vi "Configure Experiment.vi"(8 "Error In":errorcluster, 9 "KH":T4 {"KH #" items=["A 1", "A 2", "A 3", "A 4", "A 5", "A 6", "A 7", "A 8"]}, 10 "Lockin":T6 {"Label" items=["", "I+", "I-", "V1+", "V1-", "V2+", "V2-", "V3+", "V3-", "V4+", "V4-", "dV1", "dV2", "dV3", "Vsg", "Vbg", "Vtg"]}) -> (0 "Error Out":errorcluster)   [LabVIEW 2019, in "Control Experiment.lvclass"]
doc: "Use this VI to help configure your experiment.\n1. Configure the Electrode control to show which electrode is connected to which lockin channel;\n2. Choose a Label for each electrode to configure Krohn Hite amplifier automatically\n3. Easily set all Krohn Hite channels to be \"all ground\" or \"all differential\" mode\n4. Fill out information about you and your device in the lower left corner\n5. When you are finished, or when you want to update the amplifiers, click the \"CREATE OUTPUT\" button located in upper right. Clicking this button will set the amplifiers, and write information to a functional global variable that you can easily read from elsewhere in your program"
uses:
  Control Experiment.lvclass
  Typedefs/KH Mode-enum.ctl
  <userlib>/LevyLab/Krohn Hite 7008/KH7008/typedefs/Input--Enum.ctl
  <userlib>/LevyLab/Krohn Hite 7008/KH7008/typedefs/gain--enum.ctl
  <userlib>/LevyLab/Krohn Hite 7008/KH7008/typedefs/shunt--enum.ctl
  <userlib>/LevyLab/Krohn Hite 7008/KH7008/typedefs/allChannelProperties--Array.ctl
  <userlib>/LevyLab/Krohn Hite 7008/KH7008/typedefs/channelProperties--Cluster.ctl
  <userlib>/LevyLab/Krohn Hite 7008/KH7008/typedefs/channel--numeric.ctl
  <userlib>/LevyLab/Krohn Hite 7008/KH7008/typedefs/couple--Enum.ctl
  <userlib>/LevyLab/Krohn Hite 7008/KH7008/typedefs/Filter--Enum.ctl
  <userlib>/LevyLab/Configuration/Configuration.lvclass
  Typedefs/UI Controls --cluster.ctl
  Typedefs/Instruments--cluster.ctl
  Typedefs/Instrument Types--enum.ctl
  Transport Server/Inst.Transport/Inst.Transport.lvclass
  C:/Program Files/National Instruments/LabVIEW 2019/vi.lib/JKI/JKI SMO/SMO/SMO.lvclass
  C:/Program Files/National Instruments/LabVIEW 2019/user.lib/LevyLab/Instrument Framework/Instrument/Instrument.lvclass
  Transport/Transport.lvclass
  Control Experiment.lvclass/Control Experiment.ctl
  <vilib>/JKI/JKI SMO/SMO/SMO.lvclass/SMO.ctl
  Transport Server/Inst.Transport/Inst.Transport.lvclass/Inst.Transport.ctl
  Typedefs/Instrument Classes--cluster.ctl
  <userlib>/LevyLab/Instrument Framework/Instrument Types/Lockin/Instrument.LockinAPI.lvclass
  <userlib>/LevyLab/Instrument Framework/Instrument Types/Amplifier/Instrument.Amplifier.lvclass
  <userlib>/LevyLab/Instrument Framework/Instrument Types/Cryostat/Instrument.Cryostat.lvclass
  <userlib>/LevyLab/Instrument Framework/Instrument Types/CBridge/Instrument.CBridge.lvclass
  <userlib>/LevyLab/Instrument Framework/Instrument Types/Delay Line/Instrument.DelayLine.lvclass
  <userlib>/LevyLab/Instrument Framework/Instrument Types/Strain/Instrument.Strain.lvclass
  <userlib>/LevyLab/Instrument Framework/Instrument Types/VNA/Instrument.VNA.lvclass
  <userlib>/LevyLab/Instrument Framework/Instrument Types/VSource/Instrument.VSource.lvclass
  <userlib>/LevyLab/Krohn Hite 7008/Inst.Krohn-Hite-7008/Inst.Krohn-Hite-7008.lvclass
  C:/Program Files/National Instruments/LabVIEW 2019/user.lib/LevyLab/Instrument Framework/Instrument Types/Amplifier/Instrument.Amplifier.lvclass
  Typedefs/Control Experiment JSON--cluster.ctl
  b06a41f5-2f73-4e7a-a8dc-a6b31f20112d.vi
  <vilib>/JKI/JKI SMO/SMO/Private/ReftoDVR--SMO.vi
  <vilib>/JDP Science/JSONtext/Variant to JSON Text.vi
  <vilib>/JDP Science/JSONtext/LVClass Serializer/JSONtext LVClass Serializer.lvclass
  <vilib>/ErrorRing/Error Ring.xnode
  <userlib>/LevyLab/Krohn Hite 7008/KH7008/KH7008.lvlib
  <vilib>/JKI/JKI SMO/SMO/SMO.lvclass
  <userlib>/LevyLab/Instrument Framework/Instrument/Instrument.lvclass
  <vilib>/JKI/JKI SMO/URI Parsing/URI.lvlib
panel:
  in  "I'm Finished Taking Data!":bool
  out "State":string
  in  "Create Output":bool
  in  "String":string
  out "Values have changed":bool=TRUE
  in  "OK":bool
  out "Control Experiment":refnum<class "Control Experiment.lvclass">
  in  "C.E.":refnum<class "Control Experiment.lvclass">
  in  "Tab Control":enum32{"Input", "Output", "Configuration"}(tab)
  out "KH S/N":string
  out "MCL S/N":string
  in  "Transport Server":bool
  in  "Open KH7008":bool
  in  "Open Lockin":bool
  out "Lockin?":bool
  out "KH?":bool
  out "Transport?":bool
  in  "KH Chassis":i32 caption="AI Channels"
  in  "Type":u16(ring) items=["AFM", "EBL", "Cryo"]
  in  "Instrument Configuration":bool
  out "Configured Instruments":string
  in  "DC Coupled":bool=TRUE
  in  "BW Filter":bool=TRUE
  in  "AO Channels":u32=8
  in  "Gain":dbl[](array[numeric])=[1.0, 1.0, 1.0, 1.0, 1.0, 1.0, 1.0, 1.0, 1.0, 1.0, 1.0, 1.0, 1.0, 1.0, 1.0, 1.0]
  in  "AI Channels":u32=8
  in  "KH Configuration":T7(radio)
  in  "Default Resistor":T3=enum."5k"
  in  "Description":string
  in  "Sample (SAXXXX)":string
  in  "Device":string
  in  "Station":u16(ring) items=["CF900", "MNK", "PPMS (sim)", "Montana", "PPMS1", "PPMS2", "PPMS3", "OptiCool", "PPMS-W-1"]
  in  "User":u16(ring) items=["Jeremy", "Patrick", "Guanglei", "Juliana", "Ranjani", "Ahmed", "Yuhao", "Pubudu", "Sayanwita", "Aswini", "Aria", "Miles", "Bohao", "Sakshi"]
  in  "non KH":T8 {"Labels 2" items=["", "I+", "I-", "V1+", "V1-", "V2+", "V2-", "V3+", "V3-", "V4+", "V4-", "dV1", "dV2", "dV3", "Vsg", "Vbg", "Vtg"]}
  out "Device Folder":path=path "D:/Data/MNK/SA40178.20210125" caption="(\\base path\\project\\device\\ )"
  in  "Path":path=path "C:/temp" caption="Path (Typ. C:\\Users\\voodoo\\Nextcloud2\\Shared\\Instrument\\)"
  out "Comments":string
  out "JSON String":string
  in  "Label Strings":string
  # "Lockin"
  # "Krohn-Hite"
  # "Other"
  # "Channel and Chassis Configuration"
  # "Device and Project Description"
  # "Instrument Configuration"
  # "Apps"
  # "Path Configuration"
  # "Instructions: This application is used to configure your experiment\n\n1. Configure the Electrode control to show which electrode is connected to which lockin\n2. Choose a Label* for each electrode to configure Krohn Hite amplifier automatically\n3. Easily set all Krohn Hite channels to be \"all ground\" or \"all differential\" mode\n4. Fill out information about you and your device in the lower left corner\n5. When you are finished, or when you want to update the amplifiers, click the \"CONFIRM\" button located in upper right. Clicking this button will set the amplifiers and write information to a file that you can easily read from elsewhere in your program\n\n*If you want to have new labels for the \"Labels\" field you can type them below. Acceptable keywords are I, Vsg, Vbg, Vtg, dV, V, along with numeric indicies and +/-. Examples: V1+, V1-, dV1"
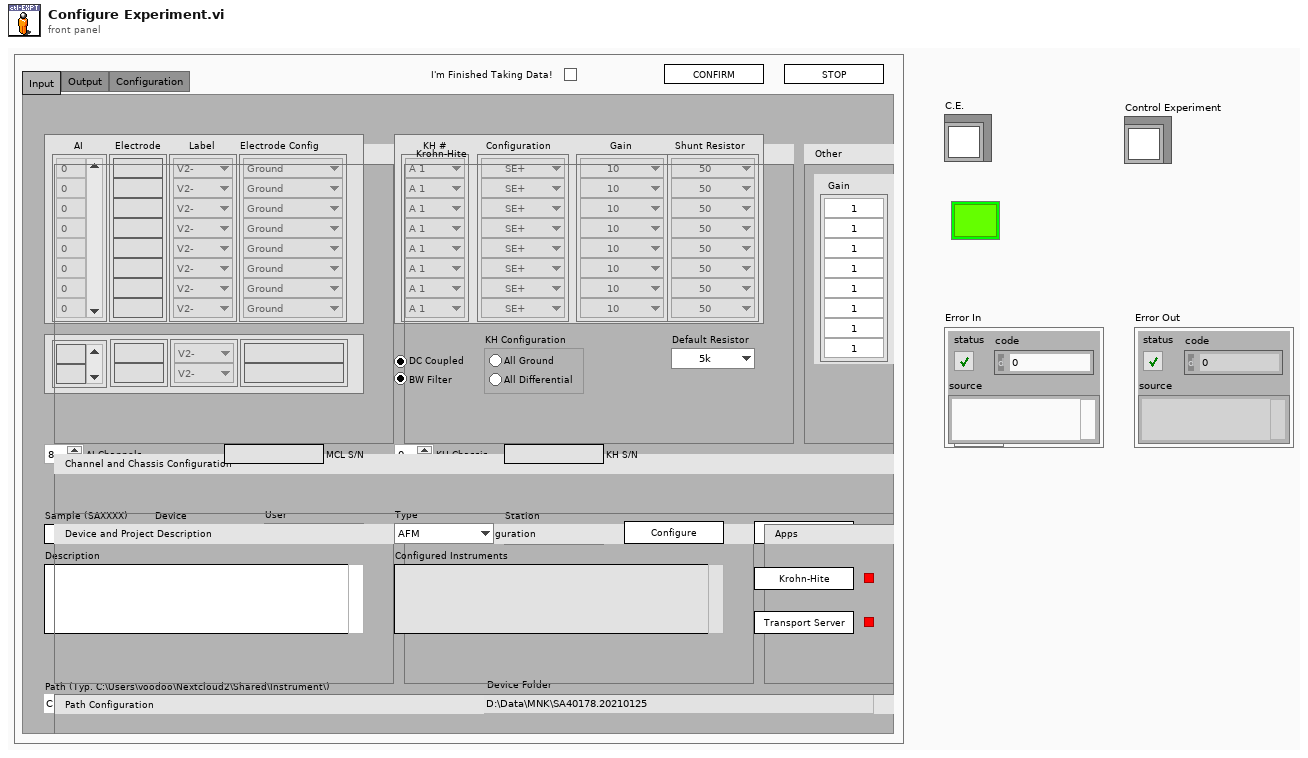
[diagram p1: front panel]
types:
  T1 = typedef "KH7008.lvlib/Input--Enum.ctl" = enum16{"OFF", "SE+", "SE-", "DIFF"}
  T2 = typedef "KH7008.lvlib/gain--enum.ctl" = enum16{"1", "10", "100", "1000"}
  T3 = typedef "KH7008.lvlib/shunt--enum.ctl" = enum16{"Open", "50", "500", "5k", "50k", "10M"}
  T4 = cluster{"KH #":u16[], "KH Configuration":T1[], "KH Gain":T2[], "KH Shunt Resistor":T3[]}
  T5 = typedef "Control Experiment.lvclass/KH Mode-enum.ctl" = enum16{"Ground", "Current", "Voltage (SE)", "Voltage (Diff)", "Gate"}
  T6 = cluster{"AI":u32[], "Electrode":string[], "Label":u16[], "Electrode Config":T5[]}
  T7 = enum32{"No Selection", "All Ground", "All Differential"}
  T8 = cluster{"Scroll Bar":string[], "Electrodes 2":string[], "Labels 2":u16[], "unused":string[]}
  T9 = enum32{"invalid app kind", "Development System", "Run Time System", "Student Edition", "Embedded LabVIEW", "Evaluation", "Custom"}
  T10 = enum32{"Bad", "Idle", "Run top level", "Running"}
  T11 = typedef "Control Experiment.lvclass/Instrument Classes--cluster.ctl" = cluster{"DAQ":refnum<class "Instrument.LockinAPI.lvclass">, "Amplifier":refnum<class "Instrument.Amplifier.lvclass">, "Temperature":refnum<class "Instrument.Cryostat.lvclass">, "Magnet":refnum<class "Instrument.Cryostat.lvclass">, "Rotator":refnum<class "Instrument.Cryostat.lvclass">, "Level":refnum<class "Instrument.Cryostat.lvclass">, "Capacitance":refnum<class "Instrument.CBridge.lvclass">, "Delay Line":refnum<class "Instrument.DelayLine.lvclass">, "Strain Cell":refnum<class "Instrument.Strain.lvclass">, "VNA":refnum<class "Instrument.VNA.lvclass">, "Source":refnum<class "Instrument.VSource.lvclass">}
  T12 = enum32{"Invalid", "Standard", "Closed", "Hidden", "Minimized", "Maximized"}
  T13 = typedef "KH7008.lvlib/channelProperties--Cluster.ctl" = cluster{"channel":T14, "gain":T2, "input":T1, "shunt":T3, "couple":T15, "filter":T16}
  T14 = typedef "KH7008.lvlib/channel--numeric.ctl" = u16
  T15 = typedef "KH7008.lvlib/couple--Enum.ctl" = enum16{"AC", "DC"}
  T16 = typedef "KH7008.lvlib/Filter--Enum.ctl" = enum16{"OFF", "ON"}
  T17 = typedef "Control Experiment.lvclass/Experiment Description--cluster.ctl" = cluster{"User":string, "Device":string, "Device Path":path, "Device Description":string, "Experiment Path":path, "Experiment Description":string, "Instrument":string, "Instruments":T18[], "Sweep":cluster{"key":string, "value":variant}[]}
  T18 = typedef "Control Experiment.lvclass/Instruments--cluster.ctl" = cluster{"class path":path, "Address":string, "Type":T19}
  T19 = typedef "Control Experiment.lvclass/Instrument Types--enum.ctl" = enum16{"DAQ", "Amplifier", "Temperature", "Magnet", "Rotator", "Level", "Capacitance", "Delay Line", "Strain Cell", "VNA", "Source"}
  T20 = typedef "Control Experiment.lvclass/Wiring Description--cluster.ctl" = cluster{"Lockin Ch":i32[], "KH":cluster{"Electrodes":string[], "Labels":string[]}, "not KH":cluster{"Electrodes":string[], "Labels":string[]}}
  T21 = typedef "KH7008.lvlib/allChannelProperties--Array.ctl" = T13[]
  T22 = typedef "Control Experiment.lvclass/UI Controls --cluster.ctl" = cluster{"Sample":string, "Device":string, "Username":string, "Description":string, "Default Path":path, "Instrument":string, "Station Type":string, "KH All Buttons":enum32{"No Selection", "All Ground", "All Differential"}, "Lockin":cluster{"AI":u32[], "Electrode":string[], "Label":u16[], "Electrode Config":T5[], "AI Channels":u32}, "KH":cluster{"KH #":enum16{"A 1", "A 2", "A 3", "A 4", "A 5", "A 6", "A 7", "A 8", "B 1", "B 2", "B 3", "B 4", "B 5", "B 6", "B 7", "B 8", "none"}[], "KH Configuration":T1[], "KH Gain":T2[], "KH Shunt Resistor":T3[], "Filter":bool, "DC Coupled":bool, "KH Chassis":i32}, "non KH":cluster{"Scroll Bar":string[], "Electrodes 2":string[], "Labels 2":u16[], "unused":string[]}, "Instrument Types":T18[]}
  T23 = cluster{"Core":cluster{"Current VI Reference":refnum<vi>, "Close Panel on Exit?":bool}, "C.E.":refnum<class "Control Experiment.lvclass">, "Experiment":T17, "Wiring Configuration":T20, "Channel Settings":cluster{"Channel Setting":T21}[], "KH Configuration":enum32{"No Selection", "All Ground", "All Differential"}, "Lockin":cluster{"AI":u32[], "Electrode":string[], "Label":u16[], "Electrode Config":T5[]}, "KH":cluster{"KH #":u16[], "KH Configuration":T1[], "KH Gain":T2[], "KH Shunt Resistor":T3[]}, "non KH":cluster{"Scroll Bar":string[], "Electrodes 2":string[], "Labels 2":u16[], "unused":string[]}, "UI":T22, "Config":refnum<class "Configuration.lvclass">, "Transport":refnum<class "Transport.lvclass">, "Transport-Server":refnum<class "Inst.Transport.lvclass">, "top level?":bool, "Instruments OK?":bool}
  T24 = typedef "SMO.lvclass/SMOState --Enum.ctl" = enum16{"unknown", "Created", "Started", "Stopped"}
  T25 = typedef "Inst.Transport.lvclass/UI State--enum.ctl" = enum16{"unknown", "Opened", "Closed"}
  T26 = cluster{"Current VI Reference":refnum<vi>, "Close Panel on Exit?":bool}
  T27 = typedef "SMO.lvclass/Public Events.ctl" = cluster{"Error":refnum<user-event>, "State":refnum<user-event>, "Reserve State":refnum<user-event>}
  T28 = typedef "Inst.Transport.lvclass/PublicEvents--Cluster.ctl" = cluster{"UI State":refnum<user-event>}
  T29 = cluster{"AI":u32[], "Electrode":string[], "Label":u16[], "Electrode Config":T5[], "AI Channels":u32}
  T30 = cluster{"KH #":enum16{"A 1", "A 2", "A 3", "A 4", "A 5", "A 6", "A 7", "A 8", "B 1", "B 2", "B 3", "B 4", "B 5", "B 6", "B 7", "B 8", "none"}[], "KH Configuration":T1[], "KH Gain":T2[], "KH Shunt Resistor":T3[], "Filter":bool, "DC Coupled":bool, "KH Chassis":i32}
  T31 = enum16{"A 1", "A 2", "A 3", "A 4", "A 5", "A 6", "A 7", "A 8", "B 1", "B 2", "B 3", "B 4", "B 5", "B 6", "B 7", "B 8", "none"}[]
  T32 = typedef "Control Experiment.lvclass/Control Experiment JSON--cluster.ctl" = cluster{"Device":cluster{"Device":string, "User":string, "Time":string, "Computer Name":string}, "Wiring":cluster{"Lockin Ch":u32[], "KH Electrodes":string[], "KH Labels":string[], "Other Electrodes":string[], "Other Labels":string[]}}
  T33 = typedef "Instrument.lvlib/Instrument.lvclass/Instrument.IDN--cluster.ctl" = cluster{"vendor":string, "model":string, "serial":string, "firmware":string}
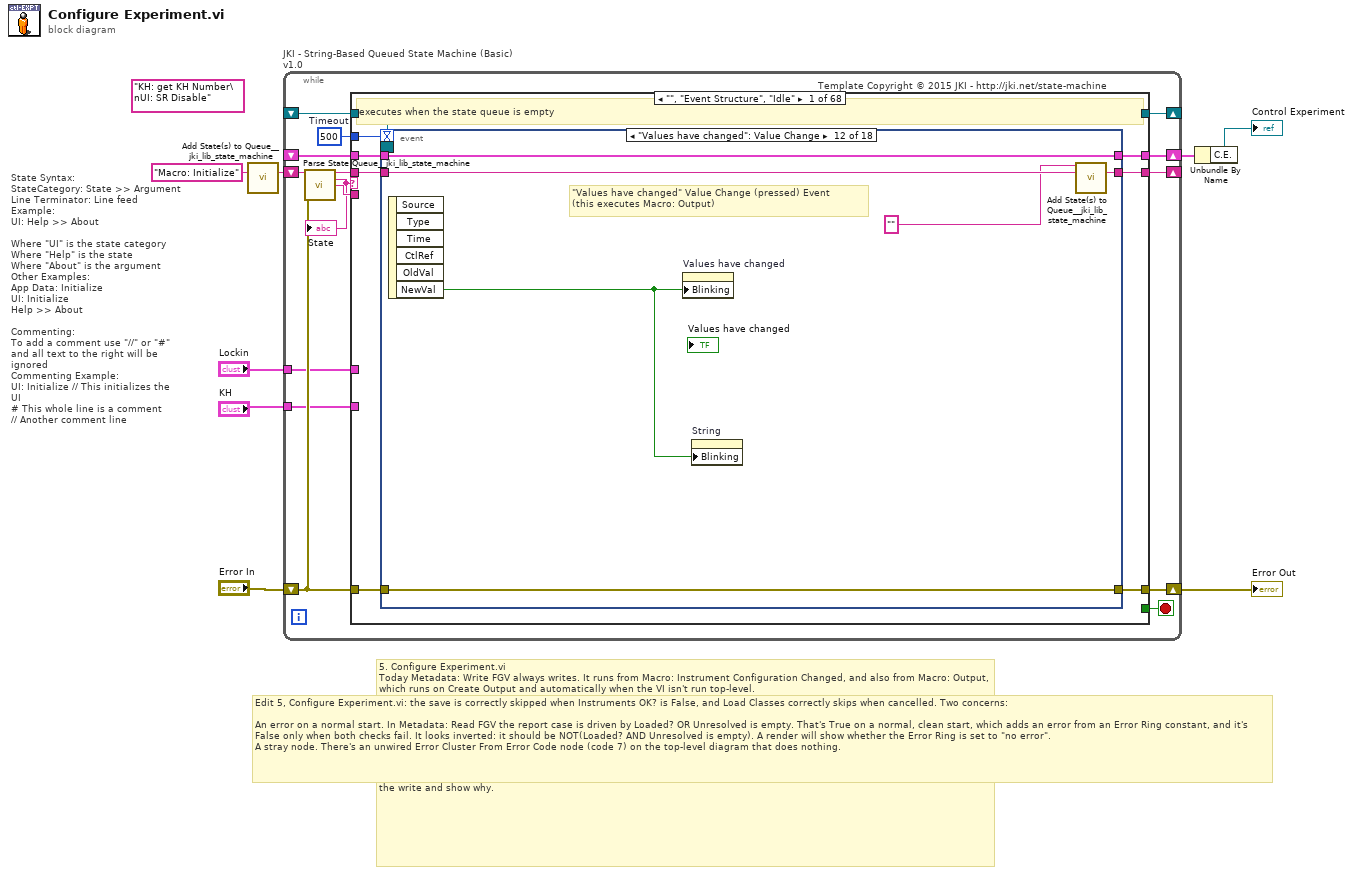
[diagram p0: block diagram]
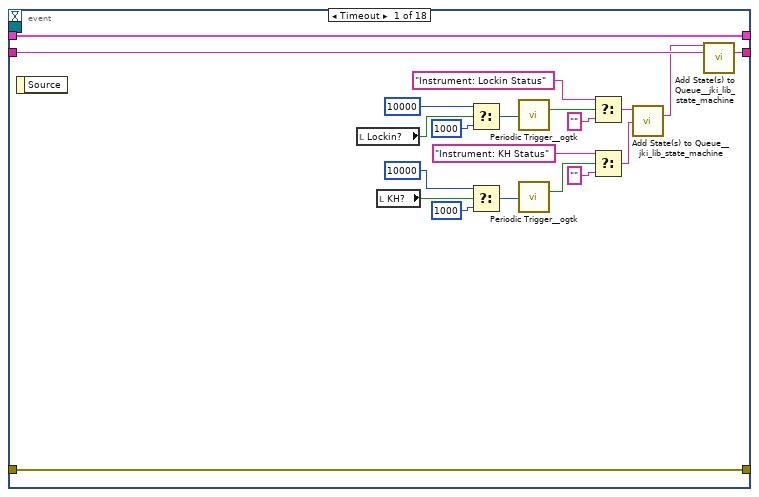
[diagram p2: hidden frame]
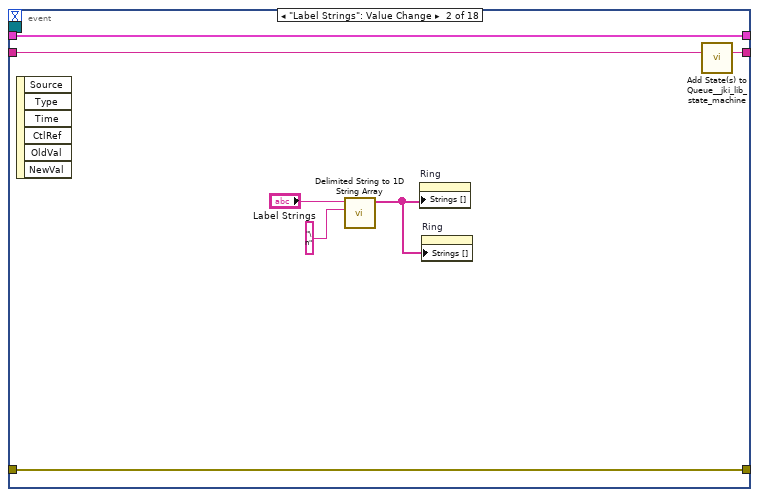
[diagram p3: hidden frame]
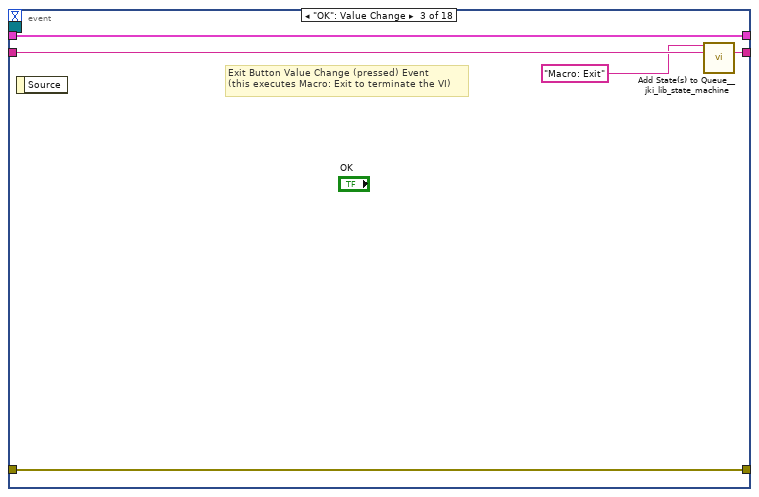
[diagram p4: hidden frame]
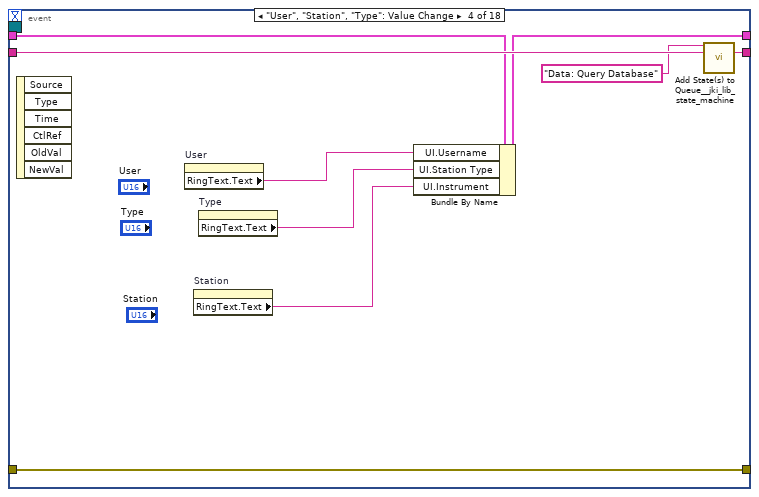
[diagram p5: hidden frame]
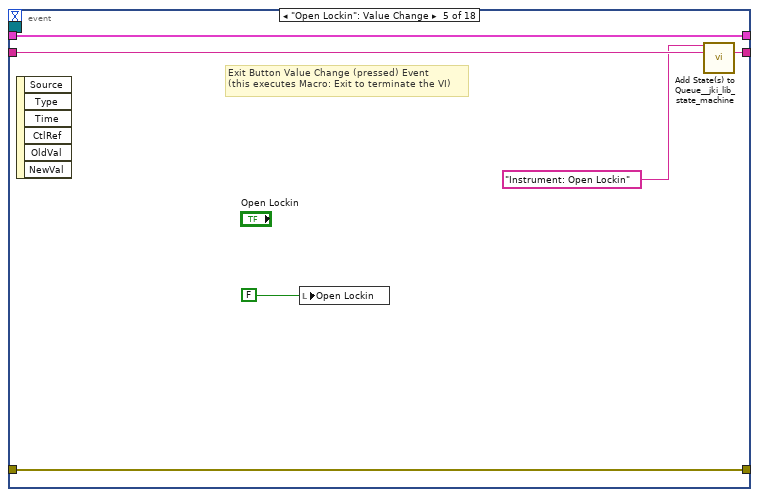
[diagram p6: hidden frame]
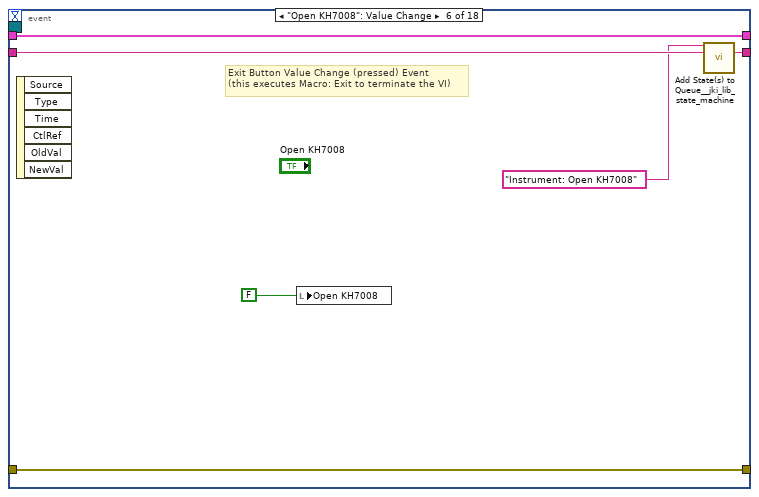
[diagram p7: hidden frame]
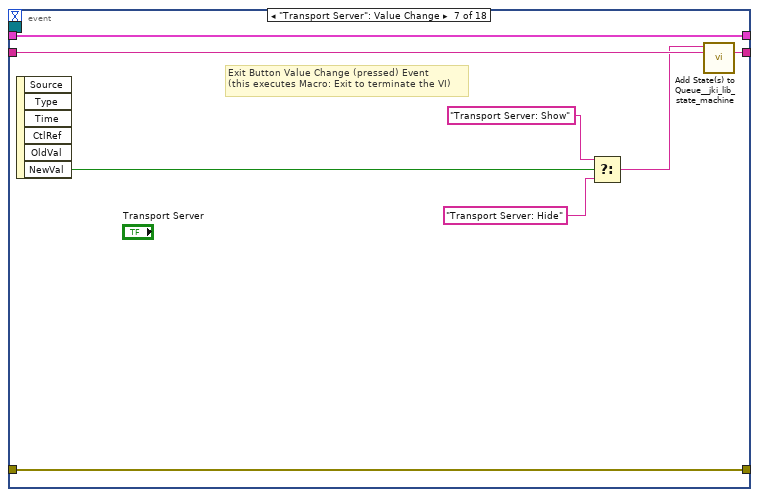
[diagram p8: hidden frame]
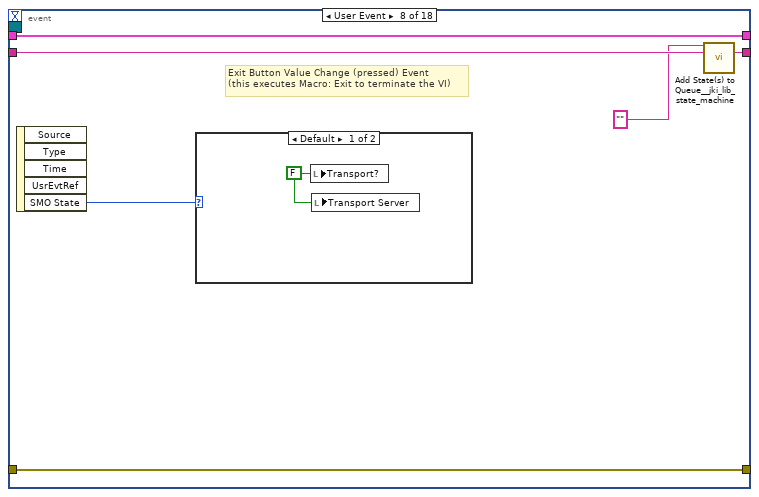
[diagram p9: hidden frame]
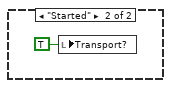
[diagram p10: hidden frame]
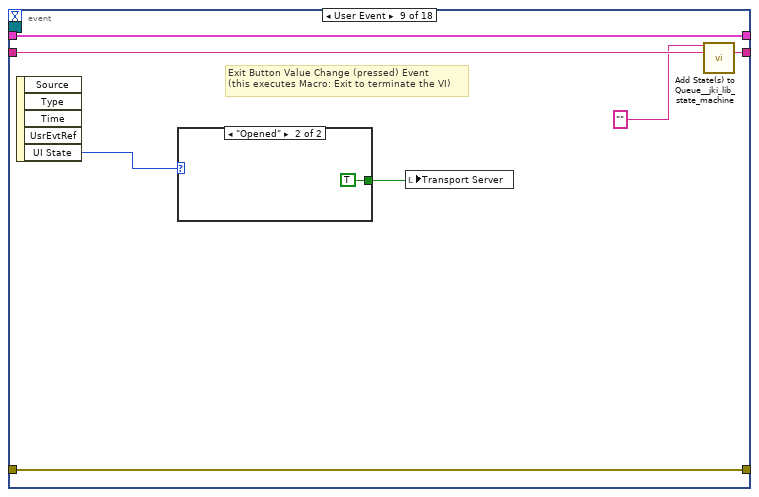
[diagram p11: hidden frame]
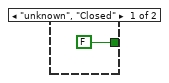
[diagram p12: hidden frame]
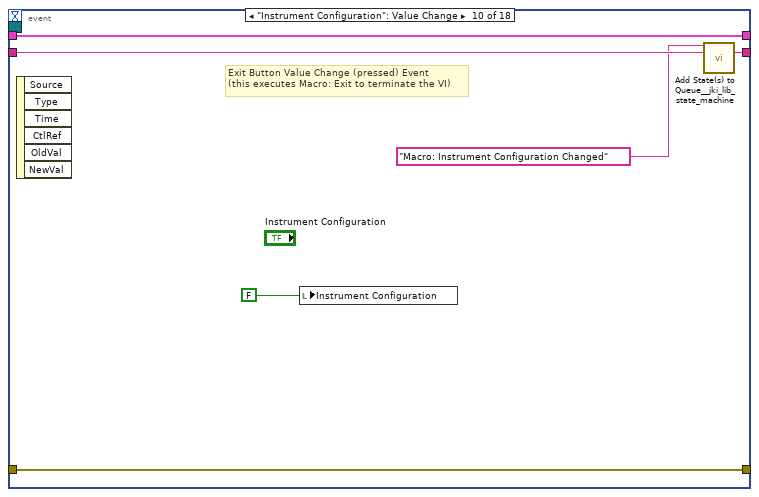
[diagram p13: hidden frame]
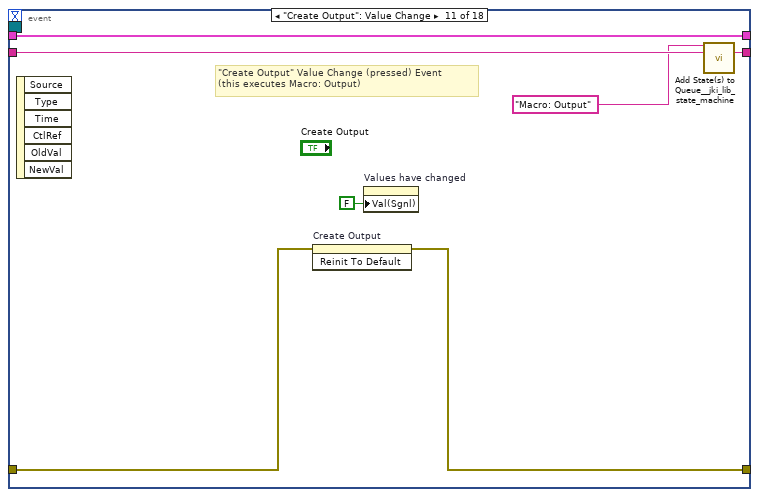
[diagram p14: hidden frame]
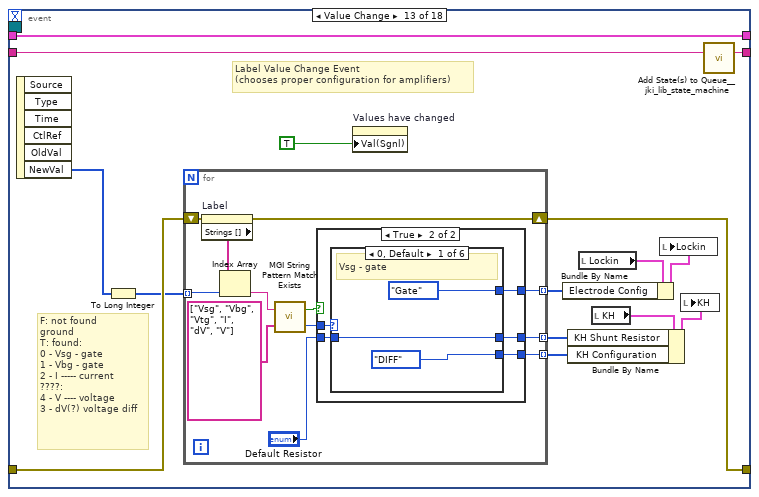
[diagram p15: hidden frame]
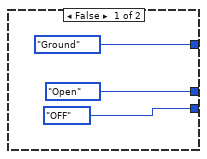
[diagram p16: hidden frame]
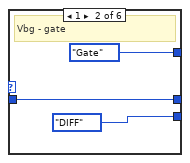
[diagram p17: hidden frame]
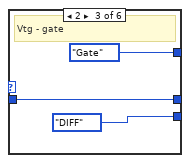
[diagram p18: hidden frame]
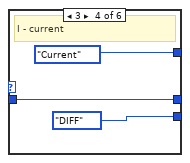
[diagram p19: hidden frame]
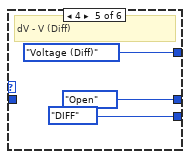
[diagram p20: hidden frame]
diagram:
  (unwired) "KH: get KH Number\nUI: SR Disable" ("State(s) in Front (\"\")")
  # "Edit 5, Configure Experiment.vi: the save is correctly skipped when Instruments OK? is False, and Load Classes correctly skips when cancelled. Two concerns:\n\nAn error on a normal start. In Metadata: Read FGV the report case is driven by Loaded? OR Unresolved is empty. That's True on a normal, clean start, which adds an error from an Error Ring constant, and it's False only when both checks fail. It looks inverted: it should be NOT(Loaded? AND Unresolved is empty). A render will show whether the Error Ring is set to \"no error\".\nA stray node. There's an unwired Error Cluster From Error Code node (code 7) on the top-level diagram that does nothing."
  # "5. Configure Experiment.vi\nToday Metadata: Write FGV always writes. It runs from Macro: Instrument Configuration Changed, and also from Macro: Output, which runs on Create Output and automatically when the VI isn't run top-level.\n\n1. Add a boolean Instruments OK? to the data cluster.\n2. Metadata: Read FGV: set Instruments OK? = Loaded? AND Unresolved on load is empty. If there's no saved configuration or entries are unresolved, tell the user: error 7 means \"no saved configuration\"; show other errors as they are.\n3. Instruments: Load Classes:\na. If Cancelled? is True, leave C.E. and Instruments OK? unchanged.\nb. Otherwise set Instruments OK? = Unresolved is empty.\n4. Metadata: Write FGV: put the Control Experiment FGV.vi (write) call inside a Case on Instruments OK?. When it is False, skip the write and show why."
  # "State Syntax:\nStateCategory: State >> Argument\nLine Terminator: Line feed\nExample:\nUI: Help >> About\n\nWhere \"UI\" is the state category\nWhere \"Help\" is the state\nWhere \"About\" is the argument\nOther Examples:\nApp Data: Initialize\nUI: Initialize\nHelp >> About\n\nCommenting:\nTo add a comment use \"//\" or \"#\" and all text to the right will be ignored\nCommenting Example:\nUI: Initialize // This initializes the UI\n# This whole line is a comment\n// Another comment line"
  n1 = call <vilib>:"Add State(s) to Queue__jki_lib_state_machine.vi"("State(s) in (\"\")"="Macro: Initialize") -> ("States Out"=w8:string)  [unwired: 14 in]
  n2 = while "JKI - String-Based Queued State Machine (Basic) v1.0" {
    shift-right: [w17] -> w6
    shift-left: _ -> [w16]
    shift-right: [w20] -> w2
    shift-left: "Error In" -> [w14]
    shift-right: [w19] -> _
    shift-left: w8 -> [w21]
    tunnel: "Lockin" -> [w13]
    tunnel: "KH" -> [w12]
    shift-right: [w10] -> _
    shift-left: _ -> [w9]
    stop <- w18 stop-if-true
    w15 = 500  # Timeout
    # "Template Copyright © 2015 JKI - http://jki.net/state-machine"
    n3 = call <vilib>:"Parse State Queue__jki_lib_state_machine.vi"("State Queue"=w21, "Error In (no error)"=w14) -> ("Remaining States"=w23:string, "Current State"=w11:string, "Arguments"=w22:string)  [unwired: 11 in]
    "State" <- w11
    n4 = case shown="\"\", \"Event Structure\", \"Idle\"" w11 {
      selector: w11 -> [_ _ w234 _ _ _ _ _ _ _ _ _ _ _ _ _ _ _ _ _ _ _ _ _ _ _ _ _ _ _ _ _ _ _ _ _ _ _ _ _ _ _ _ _ _ _ _ _ _ _ _ _ _ _ _ _ _ _ _ _ _ _ _ _ _ _ _ _]
      tunnel: w23 -> [w31 w232 w238 w257 w264 w270 w275 w295 w307 w323 w355 w362 w392 w397 w410 w416 w421 w443 w474 w494 w530 w542 w569 w585 w600 w621 w627 w639 w647 w654 w660 w666 w671 w684 w703 w728 w788 w841 w851 w863 w885 w893 w914 w927 w942 w976 w1068 w1113 w1134 w1150 w1161 w1172 w1191 w1227 w1255 w1287 w1293 w1298 w1309 w1318 w1327 w1336 w1344 w1352 w1357 w1373 w1378 w1386]
      tunnel: w22 -> [_ _ _ _ _ _ _ _ _ _ _ _ _ _ _ _ _ _ _ _ w525 w536 _ _ _ _ _ _ _ _ _ _ _ _ _ _ _ _ _ _ _ _ _ _ _ _ _ _ _ _ _ _ _ _ _ _ _ _ _ _ _ _ _ _ _ _ _ w1381]
      tunnel: w16 -> [w29 w229 w236 w248 w261 w268 w272 _ w302 w309 w335 w359 w384 w394 w408 w414 w418 w436 w463 w492 w528 w538 w566 w582 w598 w618 w624 w636 w645 w651 w657 w663 w668 w680 w699 w726 w786 w839 w847 w861 w871 w891 w908 w924 w940 w968 w1063 w1108 w1130 w1147 w1159 w1169 w1182 w1222 w1250 w1285 w1291 w1295 w1306 w1311 w1323 w1330 w1341 w1349 w1354 w1371 w1375 w1383]
      tunnel: [w28 w230 w240 w254 errorcluster {"status"=FALSE, "code"=0, "source"=""} ("error out") w267 w273 w292 w305 w320 w345 w360 w390 w395 w404 w411 w419 w424 w472 w487 w526 w539 w567 w583 w590 w619 w625 w637 w643 w652 w658 w664 w669 w682 w701 w719 w781 w834 w844 w854 w867 w889 w902 w925 w932 w967 w1065 w1106 w1131 w1148 w1154 w1170 w1189 w1225 w1253 w1283 w1289 w1296 w1300 w1314 w1319 w1333 w1340 w1348 w1355 w1363 w1376 w1384] -> w20
      tunnel: w14 -> [w27 w230 w239 w254 w260 w267 w273 w292 w305 w321 w346 w357 w390 w395 w403 w412 w419 w441 w472 w487 w527 w540 w567 w583 w591 w619 w625 w637 w643 w652 w658 w664 w669 w682 w701 w716 w778 w835 w844 w855 w873 w888 w911 w925 w930 w967 w1058 w1105 w1127 w1148 w1156 w1170 w1189 w1225 w1253 w1284 w1290 w1296 w1302 w1313 w1320 w1332 w1339 w1347 w1355 w1364 w1376 w1384]
      tunnel: [w30 w231 w237 w256 w263 w269 w274 w294 w306 w322 w354 w361 w391 w396 w409 w415 w420 w442 w473 w493 w529 w541 w568 w584 w599 w620 w626 w638 w646 w653 w659 w665 w670 w683 w702 w727 w787 w840 w850 w862 w884 w892 w913 w926 w941 w975 w1067 w1112 w1133 w1149 w1160 w1171 w1190 w1226 w1254 w1286 w1292 w1297 w1308 w1317 w1326 w1335 w1343 w1351 w1356 w1372 w1377 w1385] -> w19
      tunnel: [_ _ _ _ _ TRUE _ _ _ _ _ _ _ _ _ _ _ _ _ _ _ _ _ _ _ _ _ _ _ _ _ _ _ _ _ _ _ _ _ _ _ _ _ _ _ _ _ _ _ _ _ _ _ _ _ _ _ _ _ _ _ _ _ _ _ _ _ _] -> w18
      tunnel: [w26 w229 w236 w255 w261 w268 w272 w293 w301 w308 w336 w359 w385 w394 w408 w414 w418 w436 w463 w492 w528 w538 w566 w582 w598 w618 w624 w636 w645 w651 w657 w663 w668 w681 w700 w712 w772 w838 w846 w860 w872 w891 w909 w924 w939 w974 w1066 w1108 w1132 w1147 w1158 w1169 w1183 w1223 w1251 w1285 w1291 w1295 w1307 w1312 w1324 w1331 w1342 w1350 w1354 w1371 w1375 w1383] -> w17
      tunnel: w15 -> [w25 _ _ _ _ _ _ _ _ _ _ _ _ _ _ _ _ _ _ _ _ _ _ _ _ _ _ _ _ _ _ _ _ _ _ _ _ _ _ _ _ _ _ _ _ _ _ _ _ _ _ _ _ _ _ _ _ _ _ _ _ _ _ _ _ _ _ _]
      tunnel: w13 -> [_ _ _ _ _ _ _ w281 _ _ _ _ _ _ _ _ _ _ _ _ _ _ _ _ _ _ _ _ _ _ _ _ _ _ _ _ _ _ _ _ _ _ _ _ _ _ _ _ _ _ _ _ _ _ _ _ _ _ _ _ _ _ _ _ _ _ _ _]
      tunnel: w12 -> [_ _ _ _ _ _ _ w280 _ _ _ _ _ _ _ _ _ _ _ _ _ _ _ _ _ _ _ _ _ _ _ _ _ _ _ _ _ _ _ _ _ _ _ _ _ _ _ _ _ _ _ _ _ _ _ _ _ _ _ _ _ _ _ _ _ _ _ _]
      tunnel: [w24 w228 w233 w245 w258 w265 w271 w277 w296 w319 w324 w356 w363 w393 w402 w413 w417 w433 w445 w486 w524 w535 w565 w570 w597 w617 w622 w628 w640 w649 w655 w661 w667 w672 w687 w710 w771 w831 w842 w852 w864 w887 w907 w923 w928 w956 w1047 w1098 w1121 w1146 w1153 w1168 w1188 w1224 w1252 w1282 w1288 w1294 w1305 w1310 w1322 w1328 w1338 w1346 w1353 w1362 w1374 w1382] -> w10
      tunnel: w9 -> [w24 w228 w233 w245 w258 w265 w271 w277 w296 w319 w324 w356 w363 w393 _ w413 w417 w433 w445 w486 w524 w535 w565 w570 w597 w617 w622 w628 w640 w649 w655 w661 w667 w672 w687 w710 w771 w831 w842 w852 w864 w887 w907 w923 w928 w956 w1047 w1098 w1121 w1146 w1153 w1168 w1188 w1224 w1252 w1282 w1288 w1294 w1305 w1310 w1322 w1328 w1338 w1346 w1353 w1362 w1374 w1382]
      frame "", "Event Structure", "Idle" {
        # "executes when the state queue is empty"
        n5 = event shown="[11] \"Values have changed\": Value Change" {
          selector: w24 -> [_ _ _ _ _ _ _ _ _ _ _ _ _ _ _ _ _ _]
          dyn-events: _ -> [_ _ _ _ _ _ _ _ _ _ _ _ _ _ _ _ _ _]
          timeout: w25 -> [_ _ _ _ _ _ _ _ _ _ _ _ _ _ _ _ _ _]
          tunnel: w31 -> [w52 w57 w64 w73 w79 w85 w93 w99 w108 w116 w123 w129 w144 w184 w189 w207 w213 w227]
          tunnel: [w51 w59 w63 w72 w78 w84 w92 w98 w107 w115 w122 w128 w143 w184 w188 w206 w215 w226] -> w30
          tunnel: w29 -> [w49 w58 w61 w68 w76 w82 w90 w96 w105 w113 w121 w127 w142 w185 w190 w205 w216 w224]
          tunnel: [w50 w56 w62 w71 w77 w83 w91 w97 w106 w114 w118 w125 w133 w186 w191 w208 w212 w225] -> w28
          tunnel: w27 -> [w50 w56 w62 w71 w77 w83 w91 w97 w106 w114 w119 w125 w140 w186 w191 w208 w212 w225]
          tunnel: [w49 w58 w61 w69 w76 w82 w90 w96 w105 w113 w121 w127 w142 w185 w190 w205 w216 w224] -> w26
          event Timeout {
            n6 = event-data() -> ()  [unwired: 1 in, 1 out]
            n7 = local read "Lockin?"() -> (w36:bool)
            n8 = local read "KH?"() -> (w37:bool)
            n9 = Select(t=u32 10000 ("time (ms)"), s=w36, f=u32 1000) -> (s? t:f=w39:u32)
            n10 = Select(t=u32 10000 ("time (ms)"), s=w37, f=u32 1000) -> (s? t:f=w38:u32)
            n11 = call <userlib>:"Periodic Trigger__ogtk.vi"("time (ms)"=w39) -> ("Triggered"=w33:bool)  [unwired: 12 in, 2 out]
            n12 = call <userlib>:"Periodic Trigger__ogtk.vi"("time (ms)"=w38) -> ("Triggered"=w32:bool)  [unwired: 12 in, 2 out]
            n13 = Select(t="Instrument: Lockin Status", s=w33, f="") -> (s? t:f=w43:string)
            n14 = Select(t="Instrument: KH Status", s=w32, f="") -> (s? t:f=w46:string)
            n15 = call <vilib>:"Add State(s) to Queue__jki_lib_state_machine.vi"("State(s) in Front (\"\")"=w43, "State(s) at Back (\"\")"=w46) -> ("States Out"=w42:string)  [unwired: 13 in]
            n16 = call <vilib>:"Add State(s) to Queue__jki_lib_state_machine.vi"("State(s) in Front (\"\")"=w42, "State(s) in (\"\")"=w52) -> ("States Out"=w51:string)  [unwired: 13 in]
          }
          event "Label Strings": Value Change {
            n17 = event-data() -> ()  [unwired: 1 in, 6 out]
            n18 = call <vilib>:"Delimited String to 1D String Array.vi"("delimiter"="\n", "delimited string"="Label Strings") -> ("string array"=w54:string[])  [unwired: 9 in]
            n19 = property on="Ring" class="Ring (strict)"("Strings []"=w54) -> ()  [unwired: 2 in, 2 out]
            n20 = property on="Ring" class="Ring (strict)"("Strings []"=w54) -> ()  [unwired: 2 in, 2 out]
            n21 = call <vilib>:"Add State(s) to Queue__jki_lib_state_machine.vi"("State(s) in (\"\")"=w57) -> ("States Out"=w59:string)  [unwired: 14 in]
          }
          event "OK": Value Change {
            # "Exit Button Value Change (pressed) Event\n(this executes Macro: Exit to terminate the VI)"
            n22 = event-data() -> ()  [unwired: 1 in, 1 out]
            n23 = call <vilib>:"Add State(s) to Queue__jki_lib_state_machine.vi"("State(s) in Front (\"\")"="Macro: Exit", "State(s) in (\"\")"=w64) -> ("States Out"=w63:string)  [unwired: 13 in]
          }
          event "User", "Station", "Type": Value Change {
            n24 = event-data() -> ()  [unwired: 1 in, 6 out]
            n25 = property on="User" class="Ring (strict)"() -> ("RingText.Text"=w67:string)  [unwired: 2 in, 2 out]
            n26 = property on="Station" class="Ring (strict)"() -> ("RingText.Text"=w66:string)  [unwired: 2 in, 2 out]
            n27 = property on="Type" class="Ring (strict)"() -> ("RingText.Text"=w65:string)  [unwired: 2 in, 2 out]
            n28 = Bundle By Name(cluster=w68, "UI.Username"=w67, "UI.Station Type"=w65, "UI.Instrument"=w66) -> (w69:T23)
            n29 = call <vilib>:"Add State(s) to Queue__jki_lib_state_machine.vi"("State(s) in Front (\"\")"="Data: Query Database", "State(s) in (\"\")"=w73) -> ("States Out"=w72:string)  [unwired: 13 in]
          }
          event "Open Lockin": Value Change {
            # "Exit Button Value Change (pressed) Event\n(this executes Macro: Exit to terminate the VI)"
            n30 = event-data() -> ()  [unwired: 1 in, 6 out]
            n31 = local write "Open Lockin"(FALSE ("Open VI")) -> ()
            n32 = call <vilib>:"Add State(s) to Queue__jki_lib_state_machine.vi"("State(s) in Front (\"\")"="Instrument: Open Lockin", "State(s) in (\"\")"=w79) -> ("States Out"=w78:string)  [unwired: 13 in]
          }
          event "Open KH7008": Value Change {
            # "Exit Button Value Change (pressed) Event\n(this executes Macro: Exit to terminate the VI)"
            n33 = event-data() -> ()  [unwired: 1 in, 6 out]
            n34 = local write "Open KH7008"(FALSE ("Open VI")) -> ()
            n35 = call <vilib>:"Add State(s) to Queue__jki_lib_state_machine.vi"("State(s) in Front (\"\")"="Instrument: Open KH7008", "State(s) in (\"\")"=w85) -> ("States Out"=w84:string)  [unwired: 13 in]
          }
          event "Transport Server": Value Change {
            # "Exit Button Value Change (pressed) Event\n(this executes Macro: Exit to terminate the VI)"
            n36 = event-data() -> ("NewVal"=w86:bool)  [unwired: 1 in, 5 out]
            n37 = Select(t="Transport Server: Show", s=w86, f="Transport Server: Hide") -> (s? t:f=w87:string)
            n38 = call <vilib>:"Add State(s) to Queue__jki_lib_state_machine.vi"("State(s) in Front (\"\")"=w87, "State(s) in (\"\")"=w93) -> ("States Out"=w92:string)  [unwired: 13 in]
          }
          event User Event {
            # "Exit Button Value Change (pressed) Event\n(this executes Macro: Exit to terminate the VI)"
            n39 = event-data() -> ("SMO State"=w94:T24)  [unwired: 1 in, 4 out]
            n40 = case shown="Default" w94 {
              frame Default {
                w100 = FALSE ("Transport?")
                n41 = local write "Transport?"(w100) -> ()
                n42 = local write "Transport Server"(w100) -> ()
              }
              frame "Started" {
                n43 = local write "Transport?"(TRUE ("Transport?")) -> ()
              }
            }
            n44 = call <vilib>:"Add State(s) to Queue__jki_lib_state_machine.vi"("State(s) in Front (\"\")"="" ("State(s) in Front (\"\")"), "State(s) in (\"\")"=w99) -> ("States Out"=w98:string)  [unwired: 13 in]
          }
          event User Event {
            # "Exit Button Value Change (pressed) Event\n(this executes Macro: Exit to terminate the VI)"
            n45 = event-data() -> ("UI State"=w103:T25)  [unwired: 1 in, 4 out]
            n46 = case shown="\"Opened\"" w103 {
              tunnel: [FALSE ("Transport Server") TRUE ("Transport Server")] -> w102
              frame "unknown", "Closed" {
              }
              frame "Opened" {
              }
            }
            n47 = local write "Transport Server"(w102) -> ()
            n48 = call <vilib>:"Add State(s) to Queue__jki_lib_state_machine.vi"("State(s) in Front (\"\")"="" ("State(s) in Front (\"\")"), "State(s) in (\"\")"=w108) -> ("States Out"=w107:string)  [unwired: 13 in]
          }
          event "Instrument Configuration": Value Change {
            # "Exit Button Value Change (pressed) Event\n(this executes Macro: Exit to terminate the VI)"
            n49 = event-data() -> ()  [unwired: 1 in, 6 out]
            n50 = local write "Instrument Configuration"(FALSE ("Open VI")) -> ()
            n51 = call <vilib>:"Add State(s) to Queue__jki_lib_state_machine.vi"("State(s) in Front (\"\")"="Macro: Instrument Configuration Changed", "State(s) in (\"\")"=w116) -> ("States Out"=w115:string)  [unwired: 13 in]
          }
          event "Create Output": Value Change {
            # "\"Create Output\" Value Change (pressed) Event\n(this executes Macro: Output)"
            n52 = event-data() -> ()  [unwired: 1 in, 6 out]
            n53 = invoke on="Create Output" class="Bool" method="Reinit To Default"(error in=w119) -> (error out=w118:errorcluster)  [unwired: 2 in, 2 out]
            n54 = property on="Values have changed" class="Bool (strict)"("Val(Sgnl)"=FALSE ("Value (Signaling)")) -> ()  [unwired: 2 in, 2 out]
            n55 = call <vilib>:"Add State(s) to Queue__jki_lib_state_machine.vi"("State(s) in Front (\"\")"="Macro: Output", "State(s) in (\"\")"=w123) -> ("States Out"=w122:string)  [unwired: 13 in]
          }
          event "Values have changed": Value Change {
            # "\"Values have changed\" Value Change (pressed) Event\n(this executes Macro: Output)"
            n56 = event-data() -> ("NewVal"=w124:bool)  [unwired: 1 in, 5 out]
            n57 = property on="Values have changed" class="Bool (strict)"("Blinking"=w124) -> ()  [unwired: 2 in, 2 out]
            n58 = property on="String" class="Str"("Blinking"=w124) -> ()  [unwired: 2 in, 2 out]
            n59 = call <vilib>:"Add State(s) to Queue__jki_lib_state_machine.vi"("State(s) in Front (\"\")"="", "State(s) in (\"\")"=w129) -> ("States Out"=w128:string)  [unwired: 13 in]
          }
          event "Lockin.Label": Value Change {
            # "F: not found\nground\nT: found:\n0 - Vsg - gate\n1 - Vbg - gate\n2 - I ----- current\n????:\n4 - V ---- voltage\n3 - dV(?) voltage diff"
            # "Label Value Change Event\n(chooses proper configuration for amplifiers)"
            n60 = event-data() -> ("NewVal"=w141:u16[])  [unwired: 1 in, 5 out]
            n61 = To Long Integer(number=w141) -> (32bit integer=w130:i32[])
            n62 = for {
              tunnel: w130 -> [w153] mode=indexing
              tunnel: [w155] -> w137 mode=indexing
              tunnel: [w150] -> w134 mode=indexing
              tunnel: [w146] -> w135 mode=indexing
              shift-right: [w151] -> w133
              shift-left: w140 -> [w152]
              n63 = property on="Label" class="Ring (strict)"(error in=w152) -> (error out=w151:errorcluster, "Strings []"=w154:string[])  [unwired: 1 in, 1 out]
              n64 = Index Array(array=w154, index=w153) -> (element=w149:string)
              n65 = call <userlib>:"MGI String Pattern Match Exists.vi"("Patterns to Try"=string[] ["Vsg", "Vbg", "Vtg", "I", "dV", "V"], "String"=w149) -> ("Index of First Pattern Matched"=w156:i32, "Match Found"=w147:bool)
              n66 = case shown="True" w147 {
                tunnel: w156 -> [_ w164]
                tunnel: [KH_Mode-enum."Ground" ("Enum") w163] -> w155
                tunnel: [shunt--enum."Open" ("Shunt Resistor") w162] -> w150
                tunnel: [Input--Enum."OFF" ("Input Configuation") w161] -> w146
                tunnel: "Default Resistor" -> [_ w160]
                frame False {
                }
                frame True {
                  n67 = case shown="0, Default" w164 {
                    tunnel: [KH_Mode-enum."Gate" ("Enum") KH_Mode-enum."Gate" ("Enum") KH_Mode-enum."Gate" ("Enum") KH_Mode-enum."Current" ("Enum") KH_Mode-enum."Voltage (Diff)" ("Enum") KH_Mode-enum."Voltage (SE)" ("Enum")] -> w163
                    tunnel: [w165 w168 w171 w174 shunt--enum."Open" ("Shunt Resistor") shunt--enum."Open" ("Shunt Resistor")] -> w162
                    tunnel: [Input--Enum."DIFF" ("Input Configuation") Input--Enum."DIFF" ("Input Configuation") Input--Enum."DIFF" ("Input Configuation") Input--Enum."DIFF" ("Input Configuation") Input--Enum."DIFF" ("Input Configuation") Input--Enum."SE+" ("Input Configuation")] -> w161
                    tunnel: w160 -> [w165 w168 w171 w174 _ _]
                    frame 0, Default {
                      # "Vsg - gate"
                    }
                    frame 1 {
                      # "Vbg - gate"
                    }
                    frame 2 {
                      # "Vtg - gate"
                    }
                    frame 3 {
                      # "I - current"
                    }
                    frame 4 {
                      # "dV - V (Diff)"
                    }
                    frame 5 {
                      # "V - V (SE)"
                    }
                  }
                }
              }
            }
            n68 = property on="Values have changed" class="Bool (strict)"("Val(Sgnl)"=TRUE ("Values have changed")) -> ()  [unwired: 2 in, 2 out]
            n69 = local read "Lockin"() -> (w138:T6)
            n70 = Bundle By Name(cluster=w138, "Electrode Config"=w137) -> (w132:T6)
            n71 = local read "KH"() -> (w136:T4)
            n72 = Bundle By Name(cluster=w136, "KH Shunt Resistor"=w134, "KH Configuration"=w135) -> (w131:T4)
            n73 = local write "Lockin"(w132) -> ()
            n74 = local write "KH"(w131) -> ()
            n75 = call <vilib>:"Add State(s) to Queue__jki_lib_state_machine.vi"("State(s) in (\"\")"=w144) -> ("States Out"=w143:string)  [unwired: 14 in]
          }
          event "KH.KH Shunt Resistor", "KH.KH Gain", "non KH.Electrodes 2", "non KH.Labels 2", "Sample (SAXXXX)", "Description", "Lockin.Electrode": Value Change {
            n76 = event-data() -> ()  [unwired: 1 in, 6 out]
            n77 = property on="Values have changed" class="Bool (strict)"("Val(Sgnl)"=TRUE ("Values have changed")) -> ()  [unwired: 2 in, 2 out]
          }
          event "Lockin.AI", "non KH.Scroll Bar": Mouse Move; "Lockin.AI", "non KH.Scroll Bar": Mouse Wheel {
            n78 = event-data() -> ()  [unwired: 1 in, 5 out]
            n79 = call <vilib>:"Add State(s) to Queue__jki_lib_state_machine.vi"("State(s) in Front (\"\")"="UI: Link Scroll Bars" ("State(s) in Front (\"\")"), "State(s) in (\"\")"=w189) -> ("States Out"=w188:string)  [unwired: 13 in]
          }
          event "AI Channels": Value Change {
            n80 = event-data() -> ("NewVal"=w193:u32)  [unwired: 1 in, 5 out]
            n81 = To Long Integer(number=w193) -> (32bit integer=w192:i32)
            n82 = for {
              N: w192 -> [_]
              tunnel: [w211] -> w197 mode=indexing
              tunnel: [w210] -> w196 mode=indexing
              i -> [w210]
              n83 = Increment(x=w210) -> (x+1=w211:i32)
            }
            n84 = local read "Lockin"() -> (w204:T6)
            n85 = Initialize Array(1.0 ("element"), w192) -> (w200:dbl[])
            n86 = Bundle By Name(cluster=w204, "AI"=w197) -> (w203:T6)
            n87 = for {
              N: w192 -> [_]
              tunnel: [w209] -> w194 mode=indexing
              i -> [w209]
            }
            n88 = local read "KH"() -> (w199:T4)
            n89 = local write "Gain"(w200) -> ()
            n90 = control-ref of="KH #"() -> (w195:refnum<vi>)
            n91 = Bundle By Name(cluster=w199, "KH #"=w196) -> (w202:T4)
            n92 = local write "Lockin"(w203) -> ()
            n93 = local write "KH"(w202) -> ()
            n94 = property on="Property Node" class="Arr (strict)"(reference=w195, "Value"=w194) -> ()  [unwired: 1 in, 2 out]
            n95 = call <vilib>:"Add State(s) to Queue__jki_lib_state_machine.vi"("State(s) in Front (\"\")"="Metadata: Update AI\nMetadata: Update KH\nKH: set KH 0\nKH: set KH 1" ("State(s) in Front (\"\")"), "State(s) in (\"\")"=w207) -> ("States Out"=w206:string)  [unwired: 13 in]
          }
          event "KH Chassis": Value Change {
            n96 = event-data() -> ("NewVal"=w217:i32)  [unwired: 1 in, 5 out]
            n97 = local write "KH Chassis"(w217) -> ()
            n98 = call <vilib>:"Add State(s) to Queue__jki_lib_state_machine.vi"("State(s) in Front (\"\")"="Metadata: Update AI\nMetadata: Update KH\nKH: set KH 0\nKH: set KH 1" ("State(s) in Front (\"\")"), "State(s) in (\"\")"=w213) -> ("States Out"=w215:string)  [unwired: 13 in]
          }
          event Panel Close? {
            n99 = event-data() -> ()  [unwired: 1 in, 1 out]
            n100 = Two Button Dialog(message="Are you sure?") -> (T button?=w221:bool)  [unwired: 2 in]
            n101 = Select(t="Macro: Exit", s=w221, f="") -> (s? t:f=w219:string)
            n102 = event-data ("Event Filter Node")("Discard?"=TRUE) -> ()  [unwired: 1 in, 1 out]
            n103 = call <vilib>:"Add State(s) to Queue__jki_lib_state_machine.vi"("State(s) in Front (\"\")"=w219, "State(s) in (\"\")"=w227) -> ("States Out"=w226:string)  [unwired: 13 in]
          }
        }
      }
      frame "---------- Core ----------" {
        # "Do not put any code in this frame.\n(it is a separator no-op)"
        n104 = call <vilib>:"Add State(s) to Queue__jki_lib_state_machine.vi"("State(s) in (\"\")"=w232) -> ("States Out"=w231:string)  [unwired: 14 in]
      }
      frame Default {
        w243 = 42 items=["No error", "Argument error", "Memory is full", "Out of zone", "End of file", "File already open", "Generic file I/O error", "File not found", "File permission error", "Disk is full", "Duplicate path", "Too many files open", "System feature not enabled", "Resource file not found", "Cannot add resource", "Resource not found", "Image not found", "Image memory error", "Pen does not exist", "Config type invalid", "Config token not found", "Config parse error", "Config memory error", "Bad external code format", "Bad external code offset", "External code not present", "Null window", "Destroy window error", "Null menu", "Print aborted", "Bad print record", "Print driver error", "Windows error during printing", "Memory error during printing", "Print dialog error", "Generic print error", "Invalid device refnum", "Device not found", "Device parameter error", "Device unit error", "Cannot open device", "Device call aborted", "Generic error", "Cancelled by user", "Object ID too low", "Object ID too high", "Object not in heap", "Unknown heap", "Unknown object (invalid DefProc)", "Unknown object (DefProc not in table)", "Message out of range", "Invalid (null) method", "Unknown message", "Manager call not supported", "Bad address", "Network operation in progress", "Network operation timed out", "Connection is busy", "Network attribute not supported", "Network error", "Address in use", "System out of memory", "Connection aborted", "Connection refused", "Not connected", "Already connected", "Connection closed", "Initialization error (interapplication manager)", "Bad occurrence", "Wait on unbound occurrence handler", "Occurrence queue overflow", "Datalog type conflict", "Unused", "Unrecognized type (interapplication manager)", "Memory corrupt", "Failed to make temporary DLL", "Old CIN version", "Drag socket not found", "Failed to load drop-object", "Failed to register OLE object", "Failed to release OLE object", "Format specifier type mismatch", "Unknown format specifier", "Too few format specifiers", "Too many format specifiers", "Scan failed", "Newer CIN version", "Error converting to variant", "Runtime menu error", "Password tampered", "Variant attribute not found", "Incompatible variant data type", "Event data is not available", "Event Store is not present", "Occurrence is not found", "Event Queue is not created", "Event info is not available", "Refnum passed is NULL", "Error retrieving Class GUID", "Error retrieving CoClass GUID", "Error retrieving TypeLib GUID.", "Bad built application magic bytes.", "Specific driver is different from the specific driver associated with the Logical Name.", "There is no session opened to the class driver.", "Max Error", "MAX - Error with config objects", "MAX - Error loading configuration", "MAX - Group not supported"]
        # "Current State"
        # "Handle mistyped state name (developer tool)"
        # "Do not delete, rename, or modify this frame.\n(this is used to capture unhandled states and typos)"
        n105 = Format Into String(format string="Software Exception: Unhandled State \"%s\"." ("message"), error in=w239, w234) -> (resulting string=w242:string, error out=w241:errorcluster)  [unwired: 1 in]
        n106 = call <vilib>:"Error Cluster From Error Code.vi"("show call chain? (False)"=TRUE, "error in (no error)"=w241, "error message (\"\")"=w242, "error code (0)"=w243) -> ("error out"=w240:errorcluster)  [unwired: 5 in]
        n107 = call <vilib>:"Add State(s) to Queue__jki_lib_state_machine.vi"("State(s) in (\"\")"=w238) -> ("States Out"=w237:string)  [unwired: 14 in]
      }
      frame "Initialize Core Data" {
        # "originally closed?"
        # "exe?"
        # "If panel starts closed or is an EXE, then close it when we exit"
        # "Do not delete, rename, or modify this frame.\n(this is used to determine panel behavior on exit)"
        n108 = property on="Property Node" class="VI"() -> ("Front Panel.Open"=w253:bool)  [unwired: 2 in, 2 out]
        n109 = property on="Property Node" class="App"() -> ("App.Kind"=w252:T9)  [unwired: 2 in, 2 out]
        n110 = control-ref of="Current VI Reference"() -> (w246:refnum<vi>)
        n111 = Not(x=w253) -> (.not. x?=w250:bool)
        n112 = Equal?(x=w252, y=T9."Run Time System" ("Application:Kind")) -> (x = y?=w249:bool)
        n113 = Or(x=w250, y=w249) -> (x .or. y?=w247:bool)
        n114 = Bundle By Name(cluster=w248, "Core.Current VI Reference"=w246, "Core.Close Panel on Exit?"=w247) -> (w255:T23)
        n115 = call <vilib>:"Add State(s) to Queue__jki_lib_state_machine.vi"("State(s) in (\"\")"=w257) -> ("States Out"=w256:string)  [unwired: 14 in]
      }
      frame "Error Handler" {
        # "Unhandled Error -- Display it"
        # "Clear error"
        # "Handle any errors here.\nYou can also output any states to clean-up after errors occur"
        n116 = call <vilib>:"General Error Handler.vi"("error in (no error)"=w260) -> ()  [unwired: 10 in, 5 out]
        n117 = call <vilib>:"Add State(s) to Queue__jki_lib_state_machine.vi"("State(s) in Front (\"\")"="/* Post Error States", "State(s) in (\"\")"=w264) -> ("States Out"=w263:string)  [unwired: 13 in]
      }
      frame "Exit" {
        # "Do not put any code in this frame.\n(No errors that occur here will be handled.)"
        n118 = call <vilib>:"Add State(s) to Queue__jki_lib_state_machine.vi"("State(s) in (\"\")"=w270) -> ("States Out"=w269:string)  [unwired: 14 in]
      }
      frame "---------- Data ----------" {
        # "Do not put any code in this frame.\n(It is a separator no-op. You can make a copy of this frame to create a new Data frame)"
        n119 = call <vilib>:"Add State(s) to Queue__jki_lib_state_machine.vi"("State(s) in (\"\")"=w275) -> ("States Out"=w274:string)  [unwired: 14 in]
      }
      frame "Data: Initialize" {
        w276 = FALSE  # Instruments OK?
        w279 = refnum<class "Transport.lvclass"> refnum  # Transport
        w278 = refnum<class "Inst.Transport.lvclass"> refnum  # Transport-Server
        w282 = FALSE  # top level?
        w283 = T22 {"Sample"="", "Device"="", "Username"="", "Description"="", "Default Path"=path "", "Instrument"="", "Station Type"="", "KH All Buttons"=enum."No Selection", "Lockin"={"AI"=[], "Electrode"=[], "Label"=[], "Electrode Config"=[], "AI Channels"=16}, "KH"={"KH #"=[], "KH Configuration"=[], "KH Gain"=[], "KH Shunt Resistor"=[], "Filter"=FALSE, "DC Coupled"=FALSE, "KH Chassis"=16}, "non KH"={"Scroll Bar"=[], "Electrodes 2"=[], "Labels 2"=[], "unused"=[]}, "Instrument Types"=[]}  # UI
        w287 = refnum<class "Configuration.lvclass"> refnum  # Config
        w289 = cluster{"Channel Setting":T21}[] []  # Channel Settings
        w285 = T26 {"Current VI Reference"=refnum, "Close Panel on Exit?"=FALSE}  # Core
        # "Initialize the shift-register data, here.\n(data names are defined by what you wire into the bundle function)"
        n120 = Unbundle By Name("C.E.") -> ("Experiment"=w290:T17, "Wiring Configuration"=w291:T20)
        n121 = Bundle("Core"=w285, "C.E."="C.E.", "Experiment"=w290, "Wiring Configuration"=w291, "Channel Settings"=w289, "KH Configuration"="KH Configuration", "Lockin"=w281, "KH"=w280, "non KH"="non KH", "UI"=w283, "Config"=w287, "Transport"=w279, "Transport-Server"=w278, "top level?"=w282, "Instruments OK?"=w276) -> (w293:T23)  [unwired: 1 in]
        n122 = call <vilib>:"Add State(s) to Queue__jki_lib_state_machine.vi"("State(s) in (\"\")"=w295) -> ("States Out"=w294:string)  [unwired: 14 in]
      }
      frame "Data: Initialize Top Level" {
        # "Data: Initialize Top Level.\n(Sets top level? == T if Exec.State == Run top level, if not top level, automatically run Macro: Output, Macro: Exit)"
        n123 = property on="Property Node" class="VI"() -> ("Exec.State"=w304:T10)  [unwired: 2 in, 2 out]
        n124 = Equal?(x=w304, y=T10."Run top level" ("Execution:State")) -> (x = y?=w300:bool)
        n125 = Select(t="", s=w300, f="Macro: Output\nMacro: Exit") -> (s? t:f=w299:string)
        n126 = Bundle By Name(cluster=w302, "top level?"=w300) -> (w301:T23)
        n127 = call <vilib>:"Add State(s) to Queue__jki_lib_state_machine.vi"("State(s) in (\"\")"=w307, "State(s) at Back (\"\")"=w299) -> ("States Out"=w306:string)  [unwired: 13 in]
      }
      frame "Data: Load Configuration" {
        # "Data: Load Configuration\n(Load configuration from disk)"
        n128 = Unbundle By Name(w309) -> ("Config"=w318:refnum<class "Configuration.lvclass">, "UI"=w314:T22)
        n129 = call <userlib>:"Default Path.vi"("error in (no error)"=w321, "Folder Name [Application Name]"="Control Experiment" ("name or relative path"), "Configuration in"=w318) -> ("error out"=w316:errorcluster, "Configuration out"=w317:refnum<class "Configuration.lvclass">)  [unwired: 7 in]
        n130 = call <userlib>:"Read Configuration.vi"("INI Fomatted Cluster Type"=w314, "error in (no error)"=w316, "Configuration in"=w317) -> ("error out"=w315:errorcluster, "Configuration"=w312:variant, "Configuration out"=w313:refnum<class "Configuration.lvclass">)  [unwired: 6 in]
        n131 = Variant To Data(error in=w315, type=w314, Variant=w312) -> (data=w310:T22, error out=w320:errorcluster)
        n132 = Bundle By Name(cluster=w309, "Config"=w313, "UI"=w310) -> (w308:T23)
        n133 = call <vilib>:"Add State(s) to Queue__jki_lib_state_machine.vi"("State(s) in (\"\")"=w323) -> ("States Out"=w322:string)  [unwired: 14 in]
      }
      frame "Data: Save Controls" {
        # "Data: Save Controls\n(Write FP controls to UI Cluster and write to disk)"
        n134 = property on="User" class="Ring (strict)"() -> ("RingText.Text"=w328:string)  [unwired: 2 in, 2 out]
        n135 = Unbundle By Name(w335) -> ()  [unwired: 1 out]
        n136 = local read "Sample (SAXXXX)"() -> (w353:string)
        n137 = local read "AI Channels"() -> (w329:u32)
        n138 = local read "Path"() -> (w350:path)
        n139 = local read "KH Configuration"() -> (w349:T7)
        n140 = local read "KH"() -> (w343:T4)
        n141 = local read "Lockin"() -> (w334:T6)
        n142 = local read "non KH"() -> (w344:T8)
        n143 = property on="Station" class="Ring (strict)"() -> ("RingText.Text"=w327:string)  [unwired: 2 in, 2 out]
        n144 = local read "Description"() -> (w351:string)
        n145 = Unbundle By Name(w334) -> ("AI"=w333:u32[], "Electrode"=w332:string[], "Label"=w331:u16[], "Electrode Config"=w330:T5[])
        n146 = local read "Device"() -> (w352:string)
        n147 = Unbundle By Name(w343) -> ("KH #"=w342:u16[], "KH Configuration"=w339:T1[], "KH Gain"=w340:T2[], "KH Shunt Resistor"=w341:T3[])
        n148 = property on="Type" class="Ring (strict)"() -> ("RingText.Text"=w326:string)  [unwired: 2 in, 2 out]
        n149 = local read "KH Chassis"() -> (w325:i32)
        n150 = Bundle By Name(cluster=w335, "UI.Sample"=w353, "UI.Device"=w352, "UI.Username"=w328, "UI.Description"=w351, "UI.Default Path"=w350, "UI.Instrument"=w327, "UI.Station Type"=w326, "UI.KH All Buttons"=w349, "UI.Lockin.AI"=w333, "UI.Lockin.Electrode"=w332, "UI.Lockin.Label"=w331, "UI.Lockin.Electrode Config"=w330, "UI.Lockin.AI Channels"=w329, "UI.non KH"=w344, "UI.KH.KH #"=w342, "UI.KH.KH Configuration"=w339, "UI.KH.KH Gain"=w340, "UI.KH.KH Shunt Resistor"=w341, "UI.KH.Filter"="BW Filter", "UI.KH.DC Coupled"="DC Coupled", "UI.KH.KH Chassis"=w325) -> (w336:T23)
        n151 = Unbundle By Name(w336) -> ("Config"=w348:refnum<class "Configuration.lvclass">, "UI"=w347:T22)
        n152 = call <userlib>:"Write Configuration.vi"("error in (no error)"=w346, "Variant"=w347, "Configuration in"=w348) -> ("error out"=w345:errorcluster)  [unwired: 7 in, 1 out]
        n153 = call <vilib>:"Add State(s) to Queue__jki_lib_state_machine.vi"("State(s) in (\"\")"=w355) -> ("States Out"=w354:string)  [unwired: 14 in]
      }
      frame "Data: Cleanup" {
        # "Cleanup any data and references, here.\n(this is called automatically, by the Macro: Exit)"
        n154 = Unbundle By Name(w359) -> ("Core.Current VI Reference"=w358:refnum<vi>)
        n155 = Close Reference(reference=w358, error in (no error)=w357) -> (error out=w360:errorcluster)
        n156 = call <vilib>:"Add State(s) to Queue__jki_lib_state_machine.vi"("State(s) in (\"\")"=w362) -> ("States Out"=w361:string)  [unwired: 14 in]
      }
      frame "Data: Query Database" {
        # "Do not put any code in this frame.\n(It is a separator no-op. You can make a copy of this frame to create a new Data frame)"
        n157 = Unbundle By Name(w384) -> ("UI.Station Type"=w376:string, "UI.Instrument"=w368:string, "UI.Username"=w386:string)
        n158 = call "DB Get Station Type.vi"() -> ("Station Types"=w375:string[])  [unwired: 10 in, 1 out]
        n159 = Search 1D Array(1D array=w375, element=w376) -> (index of element=w377:i32)  [unwired: 1 in]
        n160 = property on="Type" class="Ring (strict)"("Strings []"=w375) -> (error out=w374:errorcluster)  [unwired: 2 in, 1 out]
        n161 = call "DB Get Current Users.vi"() -> ("Result (Rows or Columns)"=w380:string[])  [unwired: 10 in, 1 out]
        n162 = Less Than 0?(x=w377) -> (x < 0?=w379:bool)
        n163 = Select(t=0, s=w379, f=w377) -> (s? t:f=w373:i32)
        n164 = property on="User" class="Ring (strict)"("Strings []"=w380) -> ()  [unwired: 2 in, 2 out]
        n165 = property on="Type" class="Ring (strict)"(error in=w374, "Value"=w373) -> (error out=w372:errorcluster)  [unwired: 1 in, 1 out]
        n166 = property on="Type" class="Ring (strict)"(error in=w372) -> ("RingText.Text"=w364:string)  [unwired: 1 in, 2 out]
        n167 = Search 1D Array(1D array=w380, element=w386) -> (index of element=w389:i32)  [unwired: 1 in]
        n168 = Less Than 0?(x=w389) -> (x < 0?=w387:bool)
        n169 = Select(t=0, s=w387, f=w389) -> (s? t:f=w382:i32)
        n170 = call "DB Get Stations.vi"("Station Type"=w364) -> ("Stations"=w367:string[])  [unwired: 9 in, 1 out]
        n171 = property on="User" class="Ring (strict)"("Value"=w382) -> ("Strings []"=w383:string[])  [unwired: 2 in, 2 out]
        n172 = property on="Station" class="Ring (strict)"("Strings []"=w367) -> ()  [unwired: 2 in, 2 out]
        n173 = Search 1D Array(1D array=w367, element=w368) -> (index of element=w369:i32)  [unwired: 1 in]
        n174 = Index Array(array=w383, index=w382) -> (element=w381:string)
        n175 = Less Than 0?(x=w369) -> (x < 0?=w371:bool)
        n176 = Select(t=0, s=w371, f=w369) -> (s? t:f=w366:i32)
        n177 = property on="Station" class="Ring (strict)"("Strings []"=w367, "Value"=w366) -> ()  [unwired: 2 in, 2 out]
        n178 = Index Array(array=w367, index=w366) -> (element=w365:string)
        n179 = Bundle By Name(cluster=w384, "UI.Instrument"=w365, "UI.Station Type"=w364, "UI.Username"=w381) -> (w385:T23)
        n180 = call <vilib>:"Add State(s) to Queue__jki_lib_state_machine.vi"("State(s) in (\"\")"=w392) -> ("States Out"=w391:string)  [unwired: 14 in]
      }
      frame "---------- Events ----------" {
        # "Do not put any code in this frame.\n(It is a separator no-op. You can make a copy of this frame to create a new UI frame)"
        n181 = call <vilib>:"Add State(s) to Queue__jki_lib_state_machine.vi"("State(s) in (\"\")"=w397) -> ("States Out"=w396:string)  [unwired: 14 in]
      }
      frame "Events: Register" {
        # "Do not put any code in this frame.\n(It is a separator no-op. You can make a copy of this frame to create a new UI frame)"
        n182 = Unbundle By Name(w408) -> ("Transport-Server"=w407:refnum<class "Inst.Transport.lvclass">)
        n183 = call <vilib>:"GetPublicEvents.vi"("SMO"=w407) -> ("error out"=w398:errorcluster, "Public Events"=w406:T27, "SMO out"=w401:refnum<class "Inst.Transport.lvclass">)  [unwired: 8 in]
        n184 = call "Inst.Transport.GetPublicEvents.vi"("Inst.Transport in"=w401) -> ("error out"=w399:errorcluster, "Transport Public Events"=w400:T28)  [unwired: 8 in, 1 out]
        n185 = register-events(w406, w400) -> (reference out=w402:refnum<event-registration>, error out=w405:errorcluster)  [unwired: 2 in]
        n186 = Merge Errors(w405, w399, w398, w403) -> (w404:errorcluster)
        n187 = call <vilib>:"Add State(s) to Queue__jki_lib_state_machine.vi"("State(s) in (\"\")"=w410) -> ("States Out"=w409:string)  [unwired: 14 in]
      }
      frame "Events: Unregister" {
        # "Do not put any code in this frame.\n(It is a separator no-op. You can make a copy of this frame to create a new UI frame)"
        n188 = Unregister For Events(event registration refnum=w413, error in=w412) -> (error out=w411:errorcluster)
        n189 = call <vilib>:"Add State(s) to Queue__jki_lib_state_machine.vi"("State(s) in (\"\")"=w416) -> ("States Out"=w415:string)  [unwired: 14 in]
      }
      frame "---------- UI ----------" {
        # "Do not put any code in this frame.\n(It is a separator no-op. You can make a copy of this frame to create a new UI frame)"
        n190 = call <vilib>:"Add State(s) to Queue__jki_lib_state_machine.vi"("State(s) in (\"\")"=w421) -> ("States Out"=w420:string)  [unwired: 14 in]
      }
      frame "UI: Initialize" {
        w422 = "" ("MCL S/N")
        w432 = FALSE ("KH?")
        # "Initialize the User Interface, here.\n(this is called automatically, by the Macro: Init)"
        n191 = call <userlib>:"Fit VI window to Largest Dec__ogtk.vi"("error in (no error)"=w441, "border spacing (2 px)"=0) -> ("error out"=w425:errorcluster)  [unwired: 4 in, 1 out]
        n192 = Unbundle By Name(w436) -> ("top level?"=w435:bool)
        n193 = property on="OK" class="Bool (strict)"("Value"=FALSE ("Blinking")) -> ()  [unwired: 2 in, 2 out]
        n194 = property on="Tab Control" class="TabCtl (strict)"("Value"=enum32{"Input", "Output", "Configuration"}."Input" ("Tab Control")) -> ()  [unwired: 2 in, 2 out]
        n195 = local write "KH Configuration"(T7."No Selection" ("KH All Buttons")) -> ()
        n196 = property on="Values have changed" class="Bool (strict)"("Val(Sgnl)"=TRUE ("Blinking")) -> ()  [unwired: 2 in, 2 out]
        n197 = call <vilib>:"1D String Array to Delimited String.vi"("delimiter"="\n", "string array"=string[] ["", "I+", "I-", "V1+", "V1-", "V2+", "V2-", "V3+", "V3-", "V4+", "V4-", "dV1", "dV2", "dV3", "Vsg", "Vbg", "Vtg"] ("Strings [] 2")) -> ("delimited string"=w426:string)  [unwired: 9 in]
        n198 = local write "MCL S/N"(w422) -> ()
        n199 = local write "KH S/N"(w422) -> ()
        n200 = local write "Label Strings"(w426) -> ()
        n201 = case shown="True" w435 {
          frame False {
          }
          frame True {
            # "unused"
            n202 = property on="AI Channels" class="DigNum (strict)"("Val(Sgnl)"="AI Channels") -> ()  [unwired: 2 in, 2 out]
          }
        }
        n203 = call <vilib>:"Delimited String to 1D String Array.vi"("delimiter"="\n", "delimited string"=w426) -> ("string array"=w430:string[])  [unwired: 9 in]
        n204 = property on="Ring" class="Ring (strict)"("Strings []"=w430) -> (error out=w439:errorcluster)  [unwired: 2 in, 1 out]
        n205 = local write "Transport Server"(w432) -> ()
        n206 = property on="Ring" class="Ring (strict)"(error in=w439, "Strings []"=w430) -> (error out=w423:errorcluster)  [unwired: 1 in, 1 out]
        n207 = Merge Errors(w423, w425) -> (w424:errorcluster)
        n208 = call <vilib>:"Add State(s) to Queue__jki_lib_state_machine.vi"("State(s) in (\"\")"=w443) -> ("States Out"=w442:string)  [unwired: 14 in]
        "Lockin?" <- w432
        "KH?" <- w432
        "Transport?" <- w432
      }
      frame "UI: Update Controls" {
        # "UI: Update Controls\n(Update FP from UI cluster)"
        n209 = Unbundle By Name(w463) -> ("top level?"=w464:bool, "UI.Sample"=w468:string, "UI.Device"=w469:string, "UI.Description"=w470:string, "UI.Default Path"=w471:path, "UI.KH All Buttons"=w467:T7, "UI.Lockin"=w454:T29, "UI.KH"=w447:T30, "UI.non KH"=w458:T8)  [unwired: 2 out]
        n210 = local write "KH Configuration"(w467) -> ()
        n211 = local write "Sample (SAXXXX)"(w468) -> ()
        n212 = local write "Path"(w471) -> ()
        n213 = Unbundle By Name(w454) -> ("AI"=w453:u32[], "Electrode"=w449:string[], "Label"=w450:u16[], "Electrode Config"=w451:T5[], "AI Channels"=w448:u32)
        n214 = Unbundle By Name(w447) -> ("KH #"=w462:T31, "KH Configuration"=w459:T1[], "KH Gain"=w460:T2[], "KH Shunt Resistor"=w461:T3[], "Filter"=w457:bool, "DC Coupled"=w456:bool, "KH Chassis"=w446:i32)
        n215 = local write "Description"(w470) -> ()
        n216 = local write "Device"(w469) -> ()
        n217 = local read "Lockin"() -> (w455:T6)
        n218 = Bundle By Name(cluster=w455, "AI"=w453, "Electrode"=w449, "Label"=w450, "Electrode Config"=w451) -> (w452:T6)
        n219 = local read "KH"() -> (w466:T4)
        n220 = Bundle By Name(cluster=w466, "KH #"=w462, "KH Configuration"=w459, "KH Gain"=w460, "KH Shunt Resistor"=w461) -> (w465:T4)
        n221 = case shown="True" w464 {
          tunnel: w465 -> [_ w481]
          tunnel: w458 -> [_ w480]
          tunnel: w457 -> [_ w479]
          tunnel: w456 -> [_ w478]
          tunnel: w452 -> [_ w477]
          tunnel: w448 -> [_ w476]
          tunnel: w446 -> [_ w475]
          frame False {
          }
          frame True {
            n222 = local write "Lockin"(w477) -> ()
            n223 = local write "AI Channels"(w476) -> ()
            n224 = local write "KH"(w481) -> ()
            n225 = local write "DC Coupled"(w478) -> ()
            n226 = local write "non KH"(w480) -> ()
            n227 = local write "KH Chassis"(w475) -> ()
            n228 = local write "BW Filter"(w479) -> ()
          }
        }
        n229 = call <vilib>:"Add State(s) to Queue__jki_lib_state_machine.vi"("State(s) in (\"\")"=w474) -> ("States Out"=w473:string)  [unwired: 14 in]
      }
      frame "UI: View Instruments" {
        # "UI: View Instruments\n(convert Experiment.Instrument array to string)"
        n230 = Unbundle By Name(w492) -> ("C.E."=w483:refnum<class "Control Experiment.lvclass">)
        n231 = Cluster To Array(cluster=T11 {"DAQ"=refnum, "Amplifier"=refnum, "Temperature"=refnum, "Magnet"=refnum, "Rotator"=refnum, "Level"=refnum, "Capacitance"=refnum, "Delay Line"=refnum, "Strain Cell"=refnum, "VNA"=refnum, "Source"=refnum} ("Instrument Classes")) -> (array=w484:refnum<class "Instrument.lvclass">[])
        n232 = Unbundle By Name(w483) -> ("Instruments"=w491:T18[])
        n233 = for {
          tunnel: w484 -> [w500] mode=indexing
          tunnel: [w497] -> w482 mode=indexing
          tunnel: [w495] -> _
          n234 = call <vilib>:"Get LV Class Name.vi"("object"=w500) -> ("error out"=w496:errorcluster, "class name"=w498:string)  [unwired: 9 in]
          n235 = String To Path(string=w498) -> (path=w499:path)
          n236 = call <vilib>:"Get File Extension.vi"("error in (no error)"=w496, "file"=w499) -> ("error out"=w495:errorcluster, "filename without extension"=w497:string)  [unwired: 5 in, 3 out]
        }
        n237 = for {
          tunnel: w491 -> [w509] mode=indexing
          tunnel: [w507] -> w490 mode=indexing
          tunnel: w482 -> [w505]
          n238 = Unbundle By Name(w509) -> ("Type"=w508:T19, "class path"=w506:path, "Address"=w504:string)
          n239 = call <vilib>:"Get File Extension.vi"("file"=w506) -> ("filename without extension"=w502:string)  [unwired: 6 in, 4 out]
          n240 = call <vilib>:"Parse URI.vi"("URI"=w504) -> ("address"=w501:string)  [unwired: 6 in, 4 out]
          n241 = call <userlib>:"MGI String Pattern Match Exists.vi"("Patterns to Try"=w505, "String"=w502) -> ("Match Found"=w503:bool)  [unwired: 1 out]
          n242 = case shown="False" w503 {
            tunnel: w508 -> [w513 _]
            tunnel: [w512 ""] -> w507
            tunnel: w501 -> [w511 _]
            tunnel: w502 -> [w510 _]
            frame False {
              n243 = case shown="\"\"" w511 {
                selector: w511 -> [w514 _]
                tunnel: w513 -> [w517 w521]
                tunnel: w510 -> [w516 w520]
                tunnel: [w515 w519] -> w512
                frame Default {
                  n244 = Format Into String(format string="- %s: %s\n   - %s", w517, w516, w514) -> (resulting string=w515:string)  [unwired: 2 in, 1 out]
                }
                frame "" {
                  n245 = Format Into String(format string="- %s: %s", w521, w520) -> (resulting string=w519:string)  [unwired: 2 in, 1 out]
                }
              }
            }
            frame True {
            }
          }
        }
        n246 = call <vilib>:"1D String Array to Delimited String.vi"("delimiter"="\n", "string array"=w490) -> ("delimited string"=→"Configured Instruments":string)  [unwired: 9 in]
        n247 = call <vilib>:"Add State(s) to Queue__jki_lib_state_machine.vi"("State(s) in (\"\")"=w494) -> ("States Out"=w493:string)  [unwired: 14 in]
      }
      frame "UI: Cursor Set" {
        # "Argument"
        # "Set and Unset Cursor Busy.\n(Usage: \"UI: Cursor Set >> Busy|Idle\")"
        n248 = case shown="\"Idle\", Default" w525 {
          tunnel: w527 -> [w532 w534]
          tunnel: [w531 w533] -> w526
          frame "Idle", Default {
            n249 = call <vilib>:"Unset Busy.vi"("error in (no error)"=w532) -> ("error out"=w531:errorcluster)  [unwired: 10 in]
          }
          frame "Busy" {
            n250 = call <vilib>:"Set Busy.vi"("error in (no error)"=w534) -> ("error out"=w533:errorcluster)  [unwired: 9 in, 1 out]
          }
        }
        n251 = call <vilib>:"Add State(s) to Queue__jki_lib_state_machine.vi"("State(s) in (\"\")"=w530) -> ("States Out"=w529:string)  [unwired: 14 in]
      }
      frame "UI: Front Panel State" {
        # "Argument"
        # "Set Front Panel Open or Closed\n(Usage: \"UI: Front Panel State >> Open|Close\")"
        n252 = Unbundle By Name(w538) -> ("Core.Current VI Reference"=w537:refnum<vi>)
        n253 = case shown="\"Open\", Default" w536 {
          tunnel: w540 -> [w546 w559]
          tunnel: [w548 w560] -> w539
          tunnel: w537 -> [w547 w557]
          frame "Open", Default {
            n254 = property on="Property Node" class="VI"(reference=w547, error in=w546) -> (reference out=w544:refnum<vi>, error out=w545:errorcluster, "Front Panel.Open"=w543:bool)
            n255 = case shown="True" w543 {
              tunnel: [w551 w554] -> w548
              tunnel: w545 -> [w550 w554]
              tunnel: w544 -> [w549 _]
              frame False {
                n256 = invoke on="Invoke Node" class="VI" method="FP.Open"(reference=w549, error in=w550, "Activate"=TRUE, "State"=T12."Standard") -> (error out=w551:errorcluster)  [unwired: 1 in, 4 out]
              }
              frame True {
              }
            }
          }
          frame "Close" {
            n257 = property on="Property Node" class="VI"(reference=w557, error in=w559) -> (reference out=w556:refnum<vi>, error out=w558:errorcluster, "Front Panel.Open"=w555:bool)
            n258 = case shown="True" w555 {
              tunnel: [w561 w564] -> w560
              tunnel: w558 -> [w561 w563]
              tunnel: w556 -> [_ w562]
              frame False {
              }
              frame True {
                n259 = invoke on="Invoke Node" class="VI" method="FP.Close"(reference=w562, error in=w563) -> (error out=w564:errorcluster)  [unwired: 1 in, 2 out]
              }
            }
          }
        }
        n260 = call <vilib>:"Add State(s) to Queue__jki_lib_state_machine.vi"("State(s) in (\"\")"=w542) -> ("States Out"=w541:string)  [unwired: 14 in]
      }
      frame "UI: Buttons" {
        # "UI: Buttons"
        n261 = call <vilib>:"Add State(s) to Queue__jki_lib_state_machine.vi"("State(s) in (\"\")"=w569) -> ("States Out"=w568:string)  [unwired: 14 in]
      }
      frame "UI: Link Scroll Bars" {
        # "UI: Link Scroll Bars\n(Link all scroll bars of control arrays)"
        n262 = control-ref of="AI"() -> (w581:refnum<vi>)
        n263 = control-ref of="Electrode"() -> (w580:refnum<vi>)
        n264 = control-ref of="Label"() -> (w579:refnum<vi>)
        n265 = control-ref of="Electrode Config"() -> (w578:refnum<vi>)
        n266 = control-ref of="KH #"() -> (w577:refnum<vi>)
        n267 = control-ref of="KH Configuration"() -> (w576:refnum<vi>)
        n268 = control-ref of="KH Gain"() -> (w575:refnum<vi>)
        n269 = control-ref of="KH Shunt Resistor"() -> (w574:refnum<vi>)
        n270 = control-ref of="Gain"() -> (w572:refnum<vi>)
        n271 = property on="Property Node" class="Arr (strict)"(reference=w581) -> ("Index Values"=w571:u32[])  [unwired: 1 in, 2 out]
        n272 = property on="Property Node" class="Arr (strict)"(reference=w580, "Index Values"=w571) -> ()  [unwired: 1 in, 2 out]
        n273 = property on="Property Node" class="Arr (strict)"(reference=w579, "Index Values"=w571) -> ()  [unwired: 1 in, 2 out]
        n274 = property on="Property Node" class="Arr (strict)"(reference=w578, "Index Values"=w571) -> ()  [unwired: 1 in, 2 out]
        n275 = property on="Property Node" class="Arr (strict)"(reference=w577, "Index Values"=w571) -> ()  [unwired: 1 in, 2 out]
        n276 = property on="Property Node" class="Arr (strict)"(reference=w576, "Index Values"=w571) -> ()  [unwired: 1 in, 2 out]
        n277 = property on="Property Node" class="Arr (strict)"(reference=w575, "Index Values"=w571) -> ()  [unwired: 1 in, 2 out]
        n278 = property on="Property Node" class="Arr (strict)"(reference=w574, "Index Values"=w571) -> ()  [unwired: 1 in, 2 out]
        n279 = property on="Property Node" class="Arr (strict)"(reference=w572, "Index Values"=w571) -> ()  [unwired: 1 in, 2 out]
        n280 = property on="Scroll Bar" class="Arr (strict)"() -> ("Index Values"=w573:u32[])  [unwired: 2 in, 2 out]
        n281 = property on="Labels 2" class="Arr (strict)"("Index Values"=w573) -> ()  [unwired: 2 in, 2 out]
        n282 = property on="unused" class="Arr (strict)"("Index Values"=w573) -> ()  [unwired: 2 in, 2 out]
        n283 = property on="Electrodes 2" class="Arr (strict)"("Index Values"=w573) -> ()  [unwired: 2 in, 2 out]
        n284 = call <vilib>:"Add State(s) to Queue__jki_lib_state_machine.vi"("State(s) in (\"\")"=w585) -> ("States Out"=w584:string)  [unwired: 14 in]
      }
      frame "UI: SR Disable" {
        # "UI: SR Disable\n(Checks if attached KH7008 is configured with 500 or 10M shunt resistor)"
        n285 = Unbundle By Name(w598) -> ("C.E."=w593:refnum<class "Control Experiment.lvclass">)
        n286 = Unbundle By Name(w593) -> ("Amplifier"=w595:refnum<class "Instrument.Amplifier.lvclass">)
        n287 = local read "KH Chassis"() -> (w586:i32)
        n288 = To More Specific Class(target class=refnum<class "Inst.Krohn-Hite-7008.lvclass"> refnum ("Inst.KH7008.lvlib:Inst.Krohn-Hite-7008.lvclass"), reference=w595) -> (specific class reference=w594:refnum<class "Inst.Krohn-Hite-7008.lvclass">)  [unwired: 1 in, 1 out]
        n289 = for {
          N: w586 -> [_]
          tunnel: w594 -> [w611]
          tunnel: [w604] -> w592 mode=concatenating
          tunnel: w591 -> [w601]
          tunnel: [w612] -> w590
          i -> [w603]
          # "check"
          # "disable"
          n290 = Increment(x=w603) -> (x+1=w602:i32)
          n291 = call-dynamic "Inst.KH7008.Open.vi"("error in (no error)"=w601, "index"=w602, "Inst.Krohn-Hite-7008 in"=w611) -> ("error out"=w608:errorcluster, "Inst.Krohn-Hite-7008 out"=w610:refnum<class "Inst.Krohn-Hite-7008.lvclass">)  [unwired: 7 in]
          n292 = call-dynamic "Inst.KH7008.getShuntResistor.vi"("error in (no error)"=w608, "Inst.Krohn-Hite-7008 in"=w610) -> ("error out"=w607:errorcluster, "ShuntResistor"=w606:string, "Inst.Krohn-Hite-7008 out"=w609:refnum<class "Inst.Krohn-Hite-7008.lvclass">)  [unwired: 7 in]
          n293 = case shown="Default" w606 {
            tunnel: [2 5] -> w605
            frame Default {
            }
            frame "500" {
            }
          }
          n294 = call-dynamic "Close.vi"("error in (no error)"=w607, "Inst.Krohn-Hite-7008 in"=w609) -> ("error out"=w612:errorcluster)  [unwired: 8 in, 1 out]
          n295 = Build Array(w605) -> (w604:i32[])
        }
        n296 = control-ref of="Shunt Resistor"() -> (w588:refnum<vi>)
        n297 = control-ref of="Default Resistor"() -> (w589:refnum<vi>)
        n298 = Build Array(w588, w589) -> (w587:refnum<vi>[])
        n299 = for {
          tunnel: w592 -> [w616]
          tunnel: w587 -> [w615] mode=indexing
          # "disable"
          n300 = property on="Property Node" class="Enum (strict)"(reference=w615, "Disabled Items []"=w616) -> ()  [unwired: 1 in, 2 out]
        }
        n301 = call <vilib>:"Add State(s) to Queue__jki_lib_state_machine.vi"("State(s) in (\"\")"=w600) -> ("States Out"=w599:string)  [unwired: 14 in]
      }
      frame "---------- Macro ----------" {
        # "Do not put any code in this frame.\n(It is a separator no-op. You can make a copy of this frame to create a new Macro frame)"
        n302 = call <vilib>:"Add State(s) to Queue__jki_lib_state_machine.vi"("State(s) in (\"\")"=w621) -> ("States Out"=w620:string)  [unwired: 14 in]
      }
      frame "Macro: Initialize" {
        # "Instruments: Load Classes\nUI: View Instruments\nMetadata: Write FGV"
        # "Initialization Macro\n(This is called once, when the VI starts)"
        n303 = call <vilib>:"Add State(s) to Queue__jki_lib_state_machine.vi"("State(s) in Front (\"\")"="Data: Initialize\nInitialize Core Data\nUI: Initialize\nUI: Front Panel State >> Open\nTransport Server: Create\nEvents: Register\nTransport Server: Start\nData: Initialize Top Level\nData: Load Configuration\nMetadata: Read FGV\n\nUI: Update Controls\n\nUI: View Instruments\nUI: Update Controls\nData: Query Database\n\nInstrument: Lockin Status\nInstrument: KH Status", "State(s) in (\"\")"=w627) -> ("States Out"=w626:string)  [unwired: 13 in]
      }
      frame "Macro: Exit" {
        # "Exit Macro\n(This is called once, when the VI exits)"
        n304 = Unbundle By Name(w636) -> ("Core.Close Panel on Exit?"=w635:bool)
        n305 = property on="OK" class="Bool (strict)"("Value"=FALSE ("Blinking")) -> ()  [unwired: 2 in, 2 out]
        n306 = Select(t="UI: Front Panel State >> Close", s=w635, f="" ("Empty String Constant")) -> (s? t:f=w632:string)
        n307 = call <vilib>:"Add State(s) to Queue__jki_lib_state_machine.vi"("State(s) in (\"\")"=w632, "State(s) at Back (\"\")"="Data: Save Controls\nTransport Server: Stop\nTransport Server: Destroy\nData: Cleanup\nEvents: Unregister\nExit") -> ("States Out"=w630:string)  [unwired: 13 in]
        n308 = call <vilib>:"Add State(s) to Queue__jki_lib_state_machine.vi"("State(s) in Front (\"\")"=w630, "State(s) in (\"\")"=w639) -> ("States Out"=w638:string)  [unwired: 13 in]
      }
      frame "Macro: Output" {
        # "Macro: Output\n(Set KH7008, Write Metadata to FGV.JSON, Write Metadata to PGSQL (Device and User))"
        n309 = case shown="False" "I'm Finished Taking Data!" {
          tunnel: ["Macro: Initialize Metadata\nUI: SR Disable\nKH: set KH 0\nKH: set KH 1\nKH: set KH 2\nMacro: Write Metadata" ("State(s) in Front (\"\")") _] -> w644
          frame False {
          }
          frame True {
          }
        }
        n310 = call <vilib>:"Add State(s) to Queue__jki_lib_state_machine.vi"("State(s) in Front (\"\")"=w644, "State(s) in (\"\")"=w647, "State(s) at Back (\"\")"="PGSQL: Write" ("State(s) in Front (\"\")")) -> ("States Out"=w646:string)  [unwired: 12 in]
      }
      frame "Macro: Instrument Configuration Changed" {
        # "Do not put any code in this frame.\n(It is a separator no-op. You can make a copy of this frame to create a new Macro frame)"
        n311 = call <vilib>:"Add State(s) to Queue__jki_lib_state_machine.vi"("State(s) in Front (\"\")"="Instruments: Load Classes\nUI: View Instruments\nMetadata: Write FGV\nInstrument: Lockin Status\nInstrument: KH Status" ("State(s) in Front (\"\")"), "State(s) in (\"\")"=w654) -> ("States Out"=w653:string)  [unwired: 13 in]
      }
      frame "Macro: Initialize Metadata" {
        # "Macro: Initialize Metadata"
        n312 = call <vilib>:"Add State(s) to Queue__jki_lib_state_machine.vi"("State(s) in Front (\"\")"="Metadata: Update Experiment Description\nMetadata: Update Wiring Configuration\nMetadata: Update KH\nMetadata: Build Path\nMetadata: Update Control Experiment Wire" ("State(s) in Front (\"\")"), "State(s) in (\"\")"=w660) -> ("States Out"=w659:string)  [unwired: 13 in]
      }
      frame "Macro: Write Metadata" {
        # "Macro: Write Metadata"
        n313 = call <vilib>:"Add State(s) to Queue__jki_lib_state_machine.vi"("State(s) in Front (\"\")"="Metadata: Update Comments\nMetadata: Write JSON\nMetadata: Write FGV" ("State(s) in Front (\"\")"), "State(s) in (\"\")"=w666) -> ("States Out"=w665:string)  [unwired: 13 in]
      }
      frame "---------- Metadata ----------" {
        # "Do not put any code in this frame.\n(it is a separator no-op)"
        n314 = call <vilib>:"Add State(s) to Queue__jki_lib_state_machine.vi"("State(s) in (\"\")"=w671) -> ("States Out"=w670:string)  [unwired: 14 in]
      }
      frame "Metadata: Update Experiment Description" {
        n315 = property on="Station" class="Ring (strict)"() -> ("RingText.Text"=w673:string)  [unwired: 2 in, 2 out]
        n316 = property on="User" class="Ring (strict)"() -> ("RingText.Text"=w674:string)  [unwired: 2 in, 2 out]
        n317 = Concatenate Strings("Sample (SAXXXX)", "." ("string"), "Device") -> (w676:string)
        n318 = Bundle By Name(cluster=w680, "Experiment.Device"=w676, "Experiment.Device Description"="Description", "Experiment.User"=w674, "Experiment.Instrument"=w673) -> (w681:T23)
        n319 = call <vilib>:"Add State(s) to Queue__jki_lib_state_machine.vi"("State(s) in (\"\")"=w684) -> ("States Out"=w683:string)  [unwired: 14 in]
      }
      frame "Metadata: Update Wiring Configuration" {
        n320 = local read "Lockin"() -> (w696:T6)
        n321 = local read "non KH"() -> (w690:T8)
        n322 = local read "Lockin"() -> (w694:T6)
        n323 = Unbundle By Name(w690) -> ("Electrodes 2"=w689:string[], "Labels 2"=w688:u16[])
        n324 = Unbundle By Name(w696) -> ("AI"=w691:u32[], "Electrode"=w692:string[], "Label"=w695:u16[])
        n325 = Unbundle By Name(w694) -> ("Electrode Config"=w693:T5[])
        n326 = To Long Integer(number=w688) -> (32bit integer=w685:i32[])
        n327 = To Long Integer(number=w695) -> (32bit integer=w686:i32[])
        n328 = for {
          tunnel: w685 -> [w705] mode=indexing
          tunnel: [w704] -> w697 mode=indexing
          n329 = property on="Ring" class="Ring (strict)"() -> ("Strings []"=w706:string[])  [unwired: 2 in, 2 out]
          n330 = Index Array(array=w706, index=w705) -> (element=w704:string)
        }
        n331 = for {
          tunnel: w686 -> [w708] mode=indexing
          tunnel: [w707] -> w698 mode=indexing
          n332 = property on="Ring" class="Ring (strict)"() -> ("Strings []"=w709:string[])  [unwired: 2 in, 2 out]
          n333 = Index Array(array=w709, index=w708) -> (element=w707:string)
        }
        n334 = Bundle By Name(cluster=w699, "Wiring Configuration.Lockin Ch"=w691, "Wiring Configuration.KH.Electrodes"=w692, "Wiring Configuration.KH.Labels"=w698, "Wiring Configuration.not KH.Electrodes"=w689, "Wiring Configuration.not KH.Labels"=w697, "Lockin.Electrode Config"=w693) -> (w700:T23)
        n335 = call <vilib>:"Add State(s) to Queue__jki_lib_state_machine.vi"("State(s) in (\"\")"=w703) -> ("States Out"=w702:string)  [unwired: 14 in]
      }
      frame "Metadata: Update KH" {
        n336 = local read "KH"() -> (w725:T4)
        n337 = Unbundle By Name(w725) -> ("KH Gain"=w717:T2[], "KH Configuration"=w722:T1[], "KH Shunt Resistor"=w721:T3[], "KH #"=w714:u16[])
        n338 = Empty Array?(array=w714) -> (empty?=w715:bool)
        n339 = case shown="False" w715 {
          tunnel: [w738 w769] -> w724
          tunnel: w722 -> [w737 _]
          tunnel: w721 -> [w736 _]
          tunnel: [w735 w767] -> w720
          tunnel: w714 -> [w731 _]
          tunnel: [w734 w770] -> w719
          tunnel: [w733 w768] -> w718
          tunnel: w717 -> [w730 _]
          tunnel: w716 -> [w732 w770]
          tunnel: [w731 u16[] [] ("KH #")] -> w713
          frame False {
            n340 = Empty Array?(array=w730) -> (empty?=w729:bool)
            n341 = case shown="False" w729 {
              tunnel: [w753 w757] -> w738
              tunnel: w737 -> [w749 w759]
              tunnel: w736 -> [w748 w760]
              tunnel: [w747 w755] -> w735
              tunnel: [w746 w754] -> w734
              tunnel: [w745 w756] -> w733
              tunnel: w732 -> [w744 w754]
              tunnel: w730 -> [w740 w758]
              tunnel: w731 -> [w739 w761]
              frame False {
                n342 = call "Initialize KH Array.vi"("KH #"=w739, "Control in"=w740) -> ("Control out"=w752:variant)  [unwired: 9 in]
                n343 = call "Initialize KH Array.vi"("KH #"=w739, "Control in"=w749) -> ("Control out"=w751:variant)  [unwired: 9 in]
                n344 = call "Initialize KH Array.vi"("KH #"=w739, "Control in"=w748) -> ("Control out"=w750:variant)  [unwired: 9 in]
                n345 = Variant To Data(error in=w744, type=w740, Variant=w752) -> (data=w753:T2[], error out=w743:errorcluster)
                n346 = Variant To Data(error in=w744, type=w749, Variant=w751) -> (data=w745:T1[], error out=w742:errorcluster)
                n347 = Variant To Data(error in=w744, type=w748, Variant=w750) -> (data=w747:T3[], error out=w741:errorcluster)
                n348 = Merge Errors(w743, w742, w741) -> (w746:errorcluster)
              }
              frame True {
                n349 = Array Size(array=w761) -> (size(s)=w762:i32)
                n350 = Index Array(array=w759) -> (element=w764:T1)  [unwired: 1 in]
                n351 = Index Array(array=w760) -> (element=w763:T3)  [unwired: 1 in]
                n352 = Index Array(array=w758) -> (element=w765:T2)  [unwired: 1 in]
                n353 = Initialize Array(w765, w762) -> (w757:T2[])
                n354 = Initialize Array(w764, w762) -> (w756:T1[])
                n355 = Initialize Array(w763, w762) -> (w755:T3[])
              }
            }
          }
          frame True {
            w767 = T3[] [] items=["Open", "50", "500", "5k", "50k", "10M"] ("KH Shunt Resistor")
            w768 = T1[] [] items=["OFF", "SE+", "SE-", "DIFF"] ("KH Configuration")
            w769 = T2[] [] items=["1", "10", "100", "1000"] ("KH Gain")
          }
        }
        n356 = local read "KH Configuration"() -> (w723:T7)
        n357 = Bundle By Name(cluster=w726, "KH Configuration"=w723, "KH.KH Gain"=w724, "KH.KH Configuration"=w718, "KH.KH Shunt Resistor"=w720, "KH.KH #"=w713) -> (w712:T23)
        n358 = Unbundle By Name(w712) -> ("KH"=w711:T4)
        n359 = local write "KH"(w711) -> ()
        n360 = call <vilib>:"Add State(s) to Queue__jki_lib_state_machine.vi"("State(s) in (\"\")"=w728) -> ("States Out"=w727:string)  [unwired: 14 in]
      }
      frame "Metadata: Update AI" {
        n361 = local read "Lockin"() -> (w774:T6)
        n362 = Unbundle By Name(w774) -> ("Electrode"=w779:string[], "Label"=w784:u16[], "Electrode Config"=w783:T5[], "AI"=w776:u32[])
        n363 = Empty Array?(array=w776) -> (empty?=w777:bool)
        n364 = case shown="False" w777 {
          tunnel: [w798 string[] [] ("Electrode")] -> w785
          tunnel: w784 -> [w790 _]
          tunnel: w783 -> [w797 _]
          tunnel: [w796 w827] -> w782
          tunnel: w776 -> [w792 _]
          tunnel: [w791 w830] -> w781
          tunnel: [w795 u16[] [] ("Label")] -> w780
          tunnel: w779 -> [w793 _]
          tunnel: w778 -> [w794 w830]
          tunnel: [w792 u32[] [] ("AI")] -> w775
          frame False {
            n365 = Empty Array?(array=w790) -> (empty?=w789:bool)
            n366 = case shown="False" w789 {
              tunnel: [w813 w822] -> w798
              tunnel: w790 -> [w809 w823]
              tunnel: w797 -> [w808 w824]
              tunnel: [w807 w817] -> w796
              tunnel: [w806 w819] -> w795
              tunnel: w794 -> [w805 w814]
              tunnel: w793 -> [w801 w825]
              tunnel: w792 -> [w800 w816]
              tunnel: [w799 w814] -> w791
              frame False {
                n367 = call "Initialize KH Array.vi"("KH #"=w800, "Control in"=w801) -> ("Control out"=w812:variant)  [unwired: 9 in]
                n368 = call "Initialize KH Array.vi"("KH #"=w800, "Control in"=w809) -> ("Control out"=w811:variant)  [unwired: 9 in]
                n369 = call "Initialize KH Array.vi"("KH #"=w800, "Control in"=w808) -> ("Control out"=w810:variant)  [unwired: 9 in]
                n370 = Variant To Data(error in=w805, type=w801, Variant=w812) -> (data=w813:string[], error out=w804:errorcluster)
                n371 = Variant To Data(error in=w805, type=w809, Variant=w811) -> (data=w806:u16[], error out=w803:errorcluster)
                n372 = Variant To Data(error in=w805, type=w808, Variant=w810) -> (data=w807:T5[], error out=w802:errorcluster)
                n373 = Merge Errors(w804, w803, w802) -> (w799:errorcluster)
              }
              frame True {
                n374 = Array Size(array=w816) -> (size(s)=w815:i32)
                n375 = Index Array(array=w823) -> (element=w820:u16)  [unwired: 1 in]
                n376 = Index Array(array=w824) -> (element=w818:T5)  [unwired: 1 in]
                n377 = Index Array(array=w825) -> (element=w821:string)  [unwired: 1 in]
                n378 = Initialize Array(w821, w815) -> (w822:string[])
                n379 = Initialize Array(w820, w815) -> (w819:u16[])
                n380 = Initialize Array(w818, w815) -> (w817:T5[])
              }
            }
          }
          frame True {
            w827 = T1[] [] items=["OFF", "SE+", "SE-", "DIFF"] ("Electrode Config")
          }
        }
        n381 = Bundle By Name(cluster=w786, "Lockin.Electrode"=w785, "Lockin.Label"=w780, "Lockin.Electrode Config"=w782, "Lockin.AI"=w775) -> (w772:T23)
        n382 = Unbundle By Name(w772) -> ("Lockin"=w773:T6)
        n383 = local write "Lockin"(w773) -> ()
        n384 = call <vilib>:"Add State(s) to Queue__jki_lib_state_machine.vi"("State(s) in (\"\")"=w788) -> ("States Out"=w787:string)  [unwired: 14 in]
      }
      frame "Metadata: Build Path" {
        n385 = Unbundle By Name(w839) -> ("Experiment.Device"=w837:string)
        n386 = Build Path(base path="Path", name or relative path=w837) -> (appended path=w836:path)
        n387 = call <vilib>:"Create Directory Recursive.vi"("error in (no error)"=w835, "directory"=w836) -> ("error out"=w834:errorcluster, "directory copy"=w833:path)  [unwired: 3 in, 1 out]
        "Device Folder" <- w833
        n388 = Bundle By Name(cluster=w839, "Experiment.Device Path"=w833) -> (w838:T23)
        n389 = call <vilib>:"Add State(s) to Queue__jki_lib_state_machine.vi"("State(s) in (\"\")"=w841) -> ("States Out"=w840:string)  [unwired: 14 in]
      }
      frame "Metadata: Update Control Experiment Wire" {
        # "IS Control Experiment Class wire"
        # "Not on Control Experiment Class wire"
        n390 = Unbundle By Name(w847) -> ("C.E."=w845:refnum<class "Control Experiment.lvclass">, "Experiment"=w849:T17, "Wiring Configuration"=w848:T20)
        n391 = Bundle By Name(cluster=w845, "Experiment"=w849, "Wiring Configuration"=w848) -> (w843:refnum<class "Control Experiment.lvclass">)
        n392 = Bundle By Name(cluster=w847, "C.E."=w843) -> (w846:T23)
        n393 = call <vilib>:"Add State(s) to Queue__jki_lib_state_machine.vi"("State(s) in (\"\")"=w851) -> ("States Out"=w850:string)  [unwired: 14 in]
      }
      frame "Metadata: Update Comments" {
        n394 = Unbundle By Name(w861) -> ("C.E."=w857:refnum<class "Control Experiment.lvclass">)
        n395 = call "Generate Comments.vi"("error in (no error)"=w855, "Control Experiment"=w857) -> ("error out"=w853:errorcluster, "Control Experiment out"=w856:refnum<class "Control Experiment.lvclass">)  [unwired: 6 in, 1 out]
        n396 = call "Read Comments.vi"("error in (no error)"=w853, "Control Experiment in"=w856) -> ("error out"=w854:errorcluster, "Comments"=→"Comments":string, "Control Experiment out"=w858:refnum<class "Control Experiment.lvclass">)  [unwired: 7 in]
        n397 = Bundle By Name(cluster=w861, "C.E."=w858) -> (w860:T23)
        n398 = call <vilib>:"Add State(s) to Queue__jki_lib_state_machine.vi"("State(s) in (\"\")"=w863) -> ("States Out"=w862:string)  [unwired: 14 in]
      }
      frame "Metadata: Write JSON" {
        w875 = T32 {"Device"={"Device"="", "User"="", "Time"="", "Computer Name"=""}, "Wiring"={"Lockin Ch"=[], "KH Electrodes"=[], "KH Labels"=[], "Other Electrodes"=[], "Other Labels"=[]}}  # Control Experiment JSON
        n399 = Unbundle By Name(w871) -> ("C.E."=w869:refnum<class "Control Experiment.lvclass">, "Experiment.Device"=w883:string, "Experiment.User"=w874:string)
        n400 = Unbundle By Name(w871) -> ("Lockin.AI"=w882:u32[], "Wiring Configuration.KH.Electrodes"=w881:string[], "Wiring Configuration.KH.Labels"=w880:string[], "Wiring Configuration.not KH.Electrodes"=w878:string[], "Wiring Configuration.not KH.Labels"=w877:string[])
        n401 = call "Get Date Time ISO.vi"() -> ("ISO 8601 date-time string"=w876:string)  [unwired: 9 in, 2 out]
        n402 = call "Get Computer Name.vi"() -> ("name"=w879:string)  [unwired: 10 in, 1 out]
        n403 = Bundle By Name(cluster=w875, "Device.Device"=w883, "Device.User"=w874, "Device.Time"=w876, "Device.Computer Name"=w879) -> (w865:T32)
        n404 = Bundle By Name(cluster=w865, "Wiring.Lockin Ch"=w882, "Wiring.KH Electrodes"=w881, "Wiring.KH Labels"=w880, "Wiring.Other Electrodes"=w878, "Wiring.Other Labels"=w877) -> (w870:T32)
        n405 = call "To JSON Text.vim"("error in (no error)"=w873, "Anything"=w870) -> ("error out"=w867:errorcluster, "<JSON>"=w866:string)  [unwired: 8 in]
        "JSON String" <- w866
        n406 = Bundle By Name(cluster=w869, "json"=w866) -> (w868:refnum<class "Control Experiment.lvclass">)
        n407 = Bundle By Name(cluster=w871, "C.E."=w868) -> (w872:T23)
        n408 = call <vilib>:"Add State(s) to Queue__jki_lib_state_machine.vi"("State(s) in (\"\")"=w885) -> ("States Out"=w884:string)  [unwired: 14 in]
      }
      frame "Metadata: Write FGV" {
        n409 = Unbundle By Name(w891) -> ("C.E."=w890:refnum<class "Control Experiment.lvclass">, "Instruments OK?"=w886:bool)
        n410 = case shown="True" w886 {
          tunnel: w890 -> [_ w897]
          tunnel: [w894 w896] -> w889
          tunnel: w888 -> [w894 w895]
          frame False {
          }
          frame True {
            n411 = call "Control Experiment FGV.vi"("Function"=enum16{"read", "write"}."write", "error in (no error)"=w895, "Control Experiment.lvclass"=w897) -> ("error out"=w896:errorcluster)  [unwired: 5 in, 3 out]
          }
        }
        n412 = call <vilib>:"Add State(s) to Queue__jki_lib_state_machine.vi"("State(s) in (\"\")"=w893) -> ("States Out"=w892:string)  [unwired: 14 in]
      }
      frame "Metadata: Read FGV" {
        n413 = call "Control Experiment FGV.vi"("Function"=enum16{"read", "write"}."read", "error in (no error)"=w911) -> ("error out"=w900:errorcluster, "Unresolved on load"=w906:string[], "Loaded?"=w904:bool, "Control Experiment.lvclass out"=w910:refnum<class "Control Experiment.lvclass">)  [unwired: 6 in]
        n414 = Empty Array?(array=w906) -> (empty?=w903:bool)
        n415 = And(x=w904, y=w903) -> (x .and. y?=w901:bool)
        n416 = And(x=w904, y=w903) -> (x .and. y?=w905:bool)
        n417 = Not(x=w901) -> (.not. x?=w899:bool)
        n418 = case shown="True" w899 {
          tunnel: [w915 w918] -> w902
          tunnel: w900 -> [w915 w917]
          frame False {
          }
          frame True {
            n419 = xnode "Error Ring"() -> ("error out"=w916:errorcluster)
            n420 = Merge Errors(w917, w916) -> (w918:errorcluster)
          }
        }
        n421 = Bundle By Name(cluster=w908, "C.E."=w910, "Instruments OK?"=w905) -> (w909:T23)
        n422 = call <vilib>:"Add State(s) to Queue__jki_lib_state_machine.vi"("State(s) in (\"\")"=w914) -> ("States Out"=w913:string)  [unwired: 14 in]
      }
      frame "---------- KH ----------" {
        # "Do not put any code in this frame.\n(it is a separator no-op)"
        n423 = call <vilib>:"Add State(s) to Queue__jki_lib_state_machine.vi"("State(s) in (\"\")"=w927) -> ("States Out"=w926:string)  [unwired: 14 in]
      }
      frame "KH: set KH 0" {
        # "#KHChassis"
        # "initialize the Channel Settings array"
        n424 = Initialize Array(T13 {"channel"=0, "gain"=enum."10", "input"=enum."SE+", "shunt"=enum."50", "couple"=enum."DC", "filter"=enum."OFF"} ("Channel Settings"), 8 ("dimension size")) -> (w935:T13[])
        n425 = Bundle(w935) -> (w934:cluster{T13[]})  [unwired: 1 in]
        n426 = for {
          N: "KH Chassis" -> [_]
          tunnel: [w946] -> w931 mode=concatenating
          shift-right: [w944] -> w933
          shift-left: w930 -> [w945]
          i -> [w948]
          n427 = call "Number to Letter.vi"("Number"=w948) -> ("Letter"=w947:string)
          n428 = for {
            N: 8 -> [_]
            tunnel: w947 -> [w953]
            tunnel: [w952] -> w946 mode=indexing
            shift-right: [w950] -> w944
            shift-left: w945 -> [w951]
            i -> [w955]
            n429 = Increment(x=w955) -> (x+1=w949:i32)
            n430 = Format Into String(format string="%s %d", error in=w951, w953, w949) -> (resulting string=w952:string, error out=w950:errorcluster)  [unwired: 1 in]
          }
        }
        n431 = Initialize Array(w934, "KH Chassis") -> (w938:cluster{T13[]}[])
        n432 = Bundle By Name(cluster=w940, "Channel Settings"=w938) -> (w939:T23)
        n433 = property on="Ring" class="Ring (strict)"(error in=w933, "Strings []"=w931) -> (error out=w932:errorcluster)  [unwired: 1 in, 1 out]
        n434 = call <vilib>:"Add State(s) to Queue__jki_lib_state_machine.vi"("State(s) in (\"\")"=w942) -> ("States Out"=w941:string)  [unwired: 14 in]
      }
      frame "KH: set KH 1" {
        n435 = Unbundle By Name(w968) -> ("Channel Settings"=w957:cluster{"Channel Setting":T21}[], "KH.KH #"=w970:u16[], "KH.KH Gain"=w973:T2[], "Lockin.Electrode Config"=w971:T5[], "KH.KH Shunt Resistor"=w972:T3[], "KH Configuration"=w969:T7)
        n436 = local read "DC Coupled"() -> (w959:bool)
        n437 = local read "BW Filter"() -> (w958:bool)
        n438 = for {
          tunnel: w971 -> [w998] mode=indexing
          tunnel: w973 -> [w997] mode=indexing
          tunnel: w972 -> [w996] mode=indexing
          tunnel: w970 -> [w992] mode=indexing
          tunnel: [w1001] -> w964 mode=indexing
          tunnel: w969 -> [w1000]
          tunnel: [w999] -> w962 mode=indexing
          tunnel: [w995] -> w963 mode=indexing
          shift-right: [w988] -> w966
          shift-left: w957 -> [w989]
          tunnel: w959 -> [w984]
          tunnel: w958 -> [w979]
          n439 = property on="Ring" class="Ring (strict)"() -> ("Strings []"=w994:string[])  [unwired: 2 in, 2 out]
          n440 = case shown="\"No Selection\", Default" w1000 {
            tunnel: w998 -> [w1020 _ _]
            tunnel: [w1025 Input--Enum."OFF" ("Input Config") Input--Enum."DIFF" ("Input Config")] -> w995
            tunnel: w997 -> [w1024 w1043 w1046]
            tunnel: [w1023 w1043 w1046] -> w999
            tunnel: w996 -> [w1022 _ w1044]
            tunnel: [w1021 shunt--enum."Open" ("Shunt Resistor") w1044] -> w1001
            frame "No Selection", Default {
              n441 = case shown="\"Ground\", Default" w1020 {
                tunnel: [Input--Enum."OFF" ("Input Config") Input--Enum."DIFF" ("Input Config") Input--Enum."SE+" ("Input Config") Input--Enum."DIFF" ("Input Config") Input--Enum."DIFF" ("Input Config")] -> w1025
                tunnel: [shunt--enum."Open" ("Shunt Resistor") w1029 shunt--enum."Open" ("Shunt Resistor") shunt--enum."Open" ("Shunt Resistor") w1038] -> w1021
                tunnel: w1024 -> [w1026 w1030 w1033 w1037 w1039]
                tunnel: [w1026 w1030 w1033 w1037 w1039] -> w1023
                tunnel: w1022 -> [_ w1029 _ _ w1038]
                frame "Ground", Default {
                }
                frame "Current" {
                }
                frame "Voltage (SE)" {
                }
                frame "Voltage (Diff)" {
                }
                frame "Gate" {
                }
              }
            }
            frame "All Ground" {
            }
            frame "All Differential" {
            }
          }
          n442 = To Long Integer(number=w992) -> (32bit integer=w993:i32)
          n443 = Index Array(array=w994, index=w993) -> (element=w991:string)
          n444 = Select(t=couple--Enum."DC" ("Coupling"), s=w984, f=couple--Enum."AC" ("Coupling")) -> (s? t:f=w981:T15)
          n445 = Scan From String(format string="%s %d", input string=w991) -> (error out=w985:errorcluster, output 1=w987:string, output 2=w986:i32)  [unwired: 4 in, 2 out]
          n446 = Select(t=Filter--Enum."ON" ("Bandwidth Filter"), s=w979, f=Filter--Enum."OFF" ("Bandwidth Filter")) -> (s? t:f=w977:T16)
          n447 = case shown="No Error" w985 {
            tunnel: w1001 -> [w1018 _]
            tunnel: w999 -> [w1017 _]
            tunnel: w995 -> [w1016 _]
            tunnel: w989 -> [w1008 w1019]
            tunnel: [w1007 w1019] -> w988
            tunnel: w987 -> [w1006 _]
            tunnel: w986 -> [w1002 _]
            tunnel: w981 -> [w1005 _]
            tunnel: w977 -> [w1004 _]
            frame No Error {
              n448 = call "Letter to Number.vi"("Letter"=w1006) -> ("Number"=w1009:i32)
              n449 = Decrement(x=w1002) -> (x-1=w1003:i32)
              n450 = Index Array(array=w1008, index=w1009) -> (element=w1014:cluster{"Channel Setting":T21})
              n451 = Unbundle(w1014) -> ("Channel Setting"=w1013:T21)
              n452 = Index Array(array=w1013, index=w1003) -> (element=w1012:T13)
              n453 = Bundle By Name(cluster=w1012, "channel"=w1002, "gain"=w1017, "input"=w1016, "shunt"=w1018, "couple"=w1005, "filter"=w1004) -> (w1011:T13)
              n454 = Replace Array Subset(array=w1013, new element=w1011, index=w1003) -> (w1015:T21)
              n455 = Bundle("Channel Setting"=w1015) -> (w1010:cluster{"Channel Setting":T21})  [unwired: 1 in]
              n456 = Replace Array Subset(array=w1008, new element=w1010, index=w1009) -> (w1007:cluster{"Channel Setting":T21}[])
            }
            frame Error {
            }
          }
        }
        n457 = local write "KH Configuration"(T7."No Selection" ("KH All Buttons")) -> ()
        n458 = Bundle By Name(cluster=w968, "Channel Settings"=w966, "KH.KH Gain"=w962, "KH.KH Configuration"=w963, "KH.KH Shunt Resistor"=w964) -> (w974:T23)
        n459 = local read "KH"() -> (w965:T4)
        n460 = Bundle By Name(cluster=w965, "KH Gain"=w962, "KH Configuration"=w963, "KH Shunt Resistor"=w964) -> (w961:T4)
        n461 = local write "KH"(w961) -> ()
        n462 = call <vilib>:"Add State(s) to Queue__jki_lib_state_machine.vi"("State(s) in (\"\")"=w976) -> ("States Out"=w975:string)  [unwired: 14 in]
      }
      frame "KH: set KH 2" {
        # "getAllChannels"
        # "setAllChannels"
        n463 = Unbundle By Name(w1063) -> ("C.E."=w1051:refnum<class "Control Experiment.lvclass">)
        n464 = Unbundle By Name(w1063) -> ("Channel Settings"=w1053:cluster{"Channel Setting":T21}[])
        n465 = Unbundle By Name(w1051) -> ("Amplifier"=w1059:refnum<class "Instrument.Amplifier.lvclass">)
        n466 = To More Specific Class(target class=refnum<class "Inst.Krohn-Hite-7008.lvclass"> refnum ("Inst.KH7008.lvlib:Inst.Krohn-Hite-7008.lvclass"), reference=w1059) -> (specific class reference=w1057:refnum<class "Inst.Krohn-Hite-7008.lvclass">)  [unwired: 1 in, 1 out]
        n467 = for {
          tunnel: [w1079] -> w1061 mode=indexing
          tunnel: w1053 -> [w1082] mode=indexing
          tunnel: w1057 -> [w1074]
          tunnel: [w1077] -> w1055
          shift-right: [w1075] -> w1054
          shift-left: w1058 -> [w1071]
          i -> [w1070]
          n468 = Increment(x=w1070) -> (x+1=w1069:i32)
          n469 = Unbundle(w1082) -> ("Channel Setting"=w1080:T21)
          n470 = call-dynamic "Inst.KH7008.Open.vi"("error in (no error)"=w1071, "index"=w1069, "Inst.Krohn-Hite-7008 in"=w1074) -> ("error out"=w1072:errorcluster, "Inst.Krohn-Hite-7008 out"=w1073:refnum<class "Inst.Krohn-Hite-7008.lvclass">)  [unwired: 7 in]
          n471 = call-dynamic "Inst.KH7008.setAllChannels.vi"("error in (no error)"=w1072, "allChannelProperties"=w1080, "Inst.Krohn-Hite-7008 in"=w1073) -> ("error out"=w1084:errorcluster, "Inst.Krohn-Hite-7008 out"=w1083:refnum<class "Inst.Krohn-Hite-7008.lvclass">)  [unwired: 7 in]
          n472 = for {
            N: 10 -> [_]
            tunnel: w1083 -> [w1096]
            tunnel: [w1097] -> w1078
            tunnel: w1080 -> [w1091]
            tunnel: [w1085] -> w1079
            shift-right: [w1095] -> w1076
            shift-left: w1084 -> [w1089]
            i -> [w1086]
            stop <- w1090 stop-if-true
            n473 = Equal To 0?(x=w1086) -> (x = 0?=w1093:bool)
            n474 = Select(t=w1086, s=w1093, f=100) -> (s? t:f=w1087:i32)
            n475 = call <userlib>:"Wait (ms)__ogtk.vi"("error in (no error)"=w1089, "milliseconds to wait"=w1087) -> ("error out"=w1094:errorcluster)  [unwired: 8 in, 1 out]
            n476 = call-dynamic "Inst.KH7008.getAllChannels.vi"("error in (no error)"=w1094, "Inst.Krohn-Hite-7008 in"=w1096) -> ("error out"=w1095:errorcluster, "allChannelProperties"=w1088:T21, "Inst.Krohn-Hite-7008 out"=w1097:refnum<class "Inst.Krohn-Hite-7008.lvclass">)  [unwired: 7 in]
            n477 = Equal?(x=w1088, y=w1091) -> (x = y?=w1090:bool)
            n478 = Bundle("allChannelProperties"=w1088) -> (w1085:cluster{"allChannelProperties":T21})  [unwired: 1 in]
          }
          n479 = call-dynamic "Close.vi"("error in (no error)"=w1076, "Inst.Krohn-Hite-7008 in"=w1078) -> ("error out"=w1075:errorcluster, "Inst.Krohn-Hite-7008 out"=w1077:refnum<class "Inst.Krohn-Hite-7008.lvclass">)  [unwired: 8 in]
        }
        n480 = Bundle By Name(cluster=w1051, "Amplifier"=w1055) -> (w1049:refnum<class "Control Experiment.lvclass">)
        n481 = local read "Gain"() -> (w1064:dbl[])
        n482 = call "Multiply Gains.vi"("Other Gain"=w1064, "Array"=w1061) -> ("Gain x Other Gain"=w1052:dbl[])
        n483 = Unbundle By Name(w1049) -> ("DAQ"=w1056:refnum<class "Instrument.LockinAPI.lvclass">)
        n484 = call-dynamic "setInputGain.vi"("error in (no error)"=w1054, "InputGain"=w1052, "Instrument.LockinAPI in"=w1056) -> ("error out"=w1062:errorcluster, "Instrument.LockinAPI out"=w1050:refnum<class "Instrument.LockinAPI.lvclass">)  [unwired: 7 in]
        n485 = Bundle By Name(cluster=w1049, "DAQ"=w1050) -> (w1048:refnum<class "Control Experiment.lvclass">)
        n486 = Bundle By Name(cluster=w1063, "C.E."=w1048) -> (w1066:T23)
        n487 = call <vilib>:"Clear Errors.vi"("error in (no error)"=w1062) -> ("error out"=w1065:errorcluster)  [unwired: 5 in, 1 out]
        n488 = call <vilib>:"Add State(s) to Queue__jki_lib_state_machine.vi"("State(s) in (\"\")"=w1068) -> ("States Out"=w1067:string)  [unwired: 14 in]
      }
      frame "KH: get KH Number" {
        # "KH: Get KH Number\n(Check how many KH amplifiers are configured"
        n489 = Unbundle By Name(w1108) -> ("C.E."=w1107:refnum<class "Control Experiment.lvclass">)
        n490 = Unbundle By Name(w1107) -> ("Amplifier"=w1110:refnum<class "Instrument.Amplifier.lvclass">)
        n491 = To More Specific Class(target class=refnum<class "Inst.Krohn-Hite-7008.lvclass"> refnum ("Inst.KH7008.lvlib:Inst.Krohn-Hite-7008.lvclass"), reference=w1110) -> (specific class reference=w1109:refnum<class "Inst.Krohn-Hite-7008.lvclass">)  [unwired: 1 in, 1 out]
        n492 = call-dynamic "Inst.KH7008.Open.vi"("error in (no error)"=w1105, "index"=1, "Inst.Krohn-Hite-7008 in"=w1109) -> ("error out"=w1102:errorcluster, "Inst.Krohn-Hite-7008 out"=w1104:refnum<class "Inst.Krohn-Hite-7008.lvclass">)  [unwired: 7 in]
        n493 = case shown="No Error" w1102 {
          selector: w1102 -> [w1116 _]
          tunnel: w1104 -> [w1118 w1119]
          tunnel: [w1117 w1119] -> w1103
          tunnel: [w1115 _] -> w1101
          tunnel: [w1114 0 ("Number of Chassis")] -> w1099
          frame No Error {
            n494 = call-dynamic "Inst.KH7008.getChassis.vi"("error in (no error)"=w1116, "Inst.Krohn-Hite-7008 in"=w1118) -> ("error out"=w1115:errorcluster, "Number of Chassis"=w1114:i32, "Inst.Krohn-Hite-7008 out"=w1117:refnum<class "Inst.Krohn-Hite-7008.lvclass">)  [unwired: 7 in]
          }
          frame Error {
          }
        }
        n495 = local write "KH Chassis"(w1099) -> ()
        n496 = call-dynamic "Close.vi"("error in (no error)"=w1101, "Inst.Krohn-Hite-7008 in"=w1103) -> ("error out"=w1106:errorcluster)  [unwired: 8 in, 1 out]
        n497 = call <vilib>:"Add State(s) to Queue__jki_lib_state_machine.vi"("State(s) in (\"\")"=w1113) -> ("States Out"=w1112:string)  [unwired: 14 in]
      }
      frame "KH: get KH" {
        # "getAllChannels"
        # "setAllChannels"
        n498 = Unbundle By Name(w1130) -> ("C.E."=w1125:refnum<class "Control Experiment.lvclass">)
        n499 = Unbundle By Name(w1125) -> ("Amplifier"=w1128:refnum<class "Instrument.Amplifier.lvclass">)
        n500 = local read "KH Chassis"() -> (w1124:i32)
        n501 = To More Specific Class(target class=refnum<class "Inst.Krohn-Hite-7008.lvclass"> refnum ("Inst.KH7008.lvlib:Inst.Krohn-Hite-7008.lvclass"), reference=w1128) -> (specific class reference=w1126:refnum<class "Inst.Krohn-Hite-7008.lvclass">)  [unwired: 1 in, 1 out]
        n502 = for {
          N: w1124 -> [_]
          tunnel: [w1144] -> w1122 mode=indexing
          tunnel: w1126 -> [w1140]
          tunnel: w1127 -> [w1138]
          tunnel: [w1141] -> w1123
          i -> [w1137]
          n503 = Increment(x=w1137) -> (x+1=w1135:i32)
          n504 = call-dynamic "Inst.KH7008.Open.vi"("error in (no error)"=w1138, "index"=w1135, "Inst.Krohn-Hite-7008 in"=w1140) -> ("error out"=w1139:errorcluster, "Inst.Krohn-Hite-7008 out"=w1145:refnum<class "Inst.Krohn-Hite-7008.lvclass">)  [unwired: 7 in]
          n505 = call-dynamic "Inst.KH7008.getAllChannels.vi"("error in (no error)"=w1139, "Inst.Krohn-Hite-7008 in"=w1145) -> ("error out"=w1142:errorcluster, "allChannelProperties"=w1136:T21, "Inst.Krohn-Hite-7008 out"=w1143:refnum<class "Inst.Krohn-Hite-7008.lvclass">)  [unwired: 7 in]
          n506 = Bundle("allChannelProperties"=w1136) -> (w1144:cluster{"allChannelProperties":T21})  [unwired: 1 in]
          n507 = call-dynamic "Close.vi"("error in (no error)"=w1142, "Inst.Krohn-Hite-7008 in"=w1143) -> ("error out"=w1141:errorcluster)  [unwired: 8 in, 1 out]
        }
        n508 = Bundle By Name(cluster=w1130, "Channel Settings"=w1122) -> (w1132:T23)
        n509 = call <vilib>:"Clear Errors.vi"("error in (no error)"=w1123) -> ("error out"=w1131:errorcluster)  [unwired: 5 in, 1 out]
        n510 = call <vilib>:"Add State(s) to Queue__jki_lib_state_machine.vi"("State(s) in (\"\")"=w1134) -> ("States Out"=w1133:string)  [unwired: 14 in]
      }
      frame "---------- Instruments ----------" {
        # "Do not put any code in this frame.\n(it is a separator no-op)"
        n511 = call <vilib>:"Add State(s) to Queue__jki_lib_state_machine.vi"("State(s) in (\"\")"=w1150) -> ("States Out"=w1149:string)  [unwired: 14 in]
      }
      frame "Instruments: Load Classes" {
        n512 = Unbundle By Name(w1159) -> ("C.E."=w1157:refnum<class "Control Experiment.lvclass">)
        n513 = call "Load Instrument Classes.vi"("error in (no error)"=w1156, "C.E."=w1157) -> ("error out"=w1154:errorcluster, "unresolved"=w1151:string[], "cancelled"=w1152:bool, "Control Experiment"=w1155:refnum<class "Control Experiment.lvclass">)  [unwired: 6 in]
        n514 = case shown="False" w1152 {
          tunnel: w1159 -> [w1166 w1167]
          tunnel: [w1165 w1167] -> w1158
          tunnel: w1155 -> [w1164 _]
          tunnel: w1151 -> [w1162 _]
          frame False {
            n515 = Empty Array?(array=w1162) -> (empty?=w1163:bool)
            n516 = Bundle By Name(cluster=w1166, "C.E."=w1164, "Instruments OK?"=w1163) -> (w1165:T23)
          }
          frame True {
          }
        }
        n517 = call <vilib>:"Add State(s) to Queue__jki_lib_state_machine.vi"("State(s) in (\"\")"=w1161) -> ("States Out"=w1160:string)  [unwired: 14 in]
      }
      frame "---------- Instrument ----------" {
        n518 = call <vilib>:"Add State(s) to Queue__jki_lib_state_machine.vi"("State(s) in (\"\")"=w1172) -> ("States Out"=w1171:string)  [unwired: 14 in]
      }
      frame "Instrument: Lockin Status" {
        n519 = Unbundle By Name(w1182) -> ("C.E."=w1180:refnum<class "Control Experiment.lvclass">)
        n520 = Unbundle By Name(w1180) -> ("DAQ"=w1186:refnum<class "Instrument.LockinAPI.lvclass">)
        n521 = call-dynamic "Open.vi"("Instrument in"=w1186) -> ("error out"=w1187:errorcluster, "Instrument out"=w1185:refnum<class "Instrument.LockinAPI.lvclass">)  [unwired: 9 in]
        n522 = call <userlib>:"ACK.vi"("error in (no error)"=w1187, "Instrument in"=w1185) -> ("error out"=w1175:errorcluster, "ACK"=w1184:string, "Instrument out"=w1176:refnum<class "Instrument.LockinAPI.lvclass">)  [unwired: 7 in]
        n523 = case shown="Default" w1184 {
          tunnel: [w1200 w1205] -> w1181
          tunnel: w1180 -> [w1200 w1205]
          tunnel: [TRUE ("Lockin?") FALSE ("Lockin?")] -> w1179
          tunnel: [FALSE ("Lockin?") TRUE ("Lockin?")] -> w1178
          tunnel: w1176 -> [w1197 w1202]
          tunnel: w1175 -> [w1196 w1201]
          tunnel: [w1195 w1201] -> w1174
          tunnel: [w1194 w1202] -> w1173
          frame Default {
            n524 = call <userlib>:"IDN.vi"("error in (no error)"=w1196, "Instrument in"=w1197) -> ("error out"=w1195:errorcluster, "IDN"=w1193:T33, "Instrument in"=w1194:refnum<class "Instrument.LockinAPI.lvclass">)  [unwired: 7 in]
            n525 = Unbundle By Name(w1193) -> ("serial"=→"MCL S/N":string)
          }
          frame "" {
          }
        }
        n526 = call-dynamic "Close.vi"("error in (no error)"=w1174, "Instrument in"=w1173) -> ()  [unwired: 8 in, 2 out]
        n527 = property on="Lockin?" class="Bool (strict)"("Value"=w1179, "Blinking"=w1178) -> ()  [unwired: 2 in, 2 out]
        n528 = Bundle By Name(cluster=w1182, "C.E."=w1181) -> (w1183:T23)
        n529 = call <vilib>:"Add State(s) to Queue__jki_lib_state_machine.vi"("State(s) in Front (\"\")"="" ("State(s) in Front (\"\")"), "State(s) in (\"\")"=w1191) -> ("States Out"=w1190:string)  [unwired: 13 in]
      }
      frame "Instrument: KH Status" {
        n530 = Unbundle By Name(w1222) -> ("C.E."=w1217:refnum<class "Control Experiment.lvclass">)
        n531 = Unbundle By Name(w1217) -> ("Amplifier"=w1218:refnum<class "Instrument.Amplifier.lvclass">)
        n532 = To More Specific Class(target class=refnum<class "Inst.Krohn-Hite-7008.lvclass"> refnum ("Inst.KH7008.lvlib:Inst.Krohn-Hite-7008.lvclass"), reference=w1218) -> (specific class reference=w1216:refnum<class "Inst.Krohn-Hite-7008.lvclass">)  [unwired: 1 in, 1 out]
        n533 = call-dynamic "Inst.KH7008.Open.vi"("index"=1, "Inst.Krohn-Hite-7008 in"=w1216) -> ("error out"=w1207:errorcluster, "Inst.Krohn-Hite-7008 out"=w1208:refnum<class "Inst.Krohn-Hite-7008.lvclass">)  [unwired: 8 in]
        n534 = call <userlib>:"ACK.vi"("error in (no error)"=w1207, "Instrument in"=w1208) -> ("error out"=w1211:errorcluster, "ACK"=w1215:string, "Instrument out"=w1212:refnum<class "Inst.Krohn-Hite-7008.lvclass">)  [unwired: 7 in]
        n535 = case shown="Default" w1215 {
          tunnel: [w1233 w1239] -> w1221
          tunnel: w1217 -> [w1233 w1239]
          tunnel: ["" ("State(s) in Front (\"\")") "KH: get KH Number\nInstrument: get KH SN\nUI: SR Disable" ("State(s) in Front (\"\")")] -> w1220
          tunnel: [FALSE ("KH?") TRUE ("KH?")] -> w1214
          tunnel: [TRUE ("KH?") FALSE ("KH?")] -> w1213
          tunnel: w1212 -> [w1231 w1234]
          tunnel: w1211 -> [w1230 w1235]
          tunnel: [w1230 w1235] -> w1210
          tunnel: [w1231 w1234] -> w1209
          frame "" {
          }
          frame Default {
          }
        }
        n536 = property on="KH?" class="Bool (strict)"("Value"=w1214, "Blinking"=w1213) -> ()  [unwired: 2 in, 2 out]
        n537 = call-dynamic "Close.vi"("error in (no error)"=w1210, "Inst.Krohn-Hite-7008 in"=w1209) -> ()  [unwired: 8 in, 2 out]
        n538 = Bundle By Name(cluster=w1222, "C.E."=w1221) -> (w1223:T23)
        n539 = call <vilib>:"Add State(s) to Queue__jki_lib_state_machine.vi"("State(s) in Front (\"\")"=w1220, "State(s) in (\"\")"=w1227) -> ("States Out"=w1226:string)  [unwired: 13 in]
      }
      frame "Instrument: get KH SN" {
        n540 = Unbundle By Name(w1250) -> ("C.E."=w1245:refnum<class "Control Experiment.lvclass">)
        n541 = Unbundle By Name(w1245) -> ("Amplifier"=w1246:refnum<class "Instrument.Amplifier.lvclass">)
        n542 = local read "KH Chassis"() -> (w1243:i32)
        n543 = To More Specific Class(target class=refnum<class "Inst.Krohn-Hite-7008.lvclass"> refnum ("Inst.KH7008.lvlib:Inst.Krohn-Hite-7008.lvclass"), reference=w1246) -> (specific class reference=w1244:refnum<class "Inst.Krohn-Hite-7008.lvclass">)  [unwired: 1 in, 1 out]
        n544 = for {
          N: w1243 -> [_]
          tunnel: [w1267] -> w1248
          tunnel: w1244 -> [w1261]
          shift-right: [w1268] -> w1249
          shift-left: w1245 -> [w1266]
          tunnel: [w1256] -> w1242 mode=indexing
          i -> [w1258]
          n545 = Increment(x=w1258) -> (x+1=w1257:i32)
          n546 = call-dynamic "Inst.KH7008.Open.vi"("index"=w1257, "Inst.Krohn-Hite-7008 in"=w1261) -> ("error out"=w1259:errorcluster, "Inst.Krohn-Hite-7008 out"=w1260:refnum<class "Inst.Krohn-Hite-7008.lvclass">)  [unwired: 8 in]
          n547 = call <userlib>:"ACK.vi"("error in (no error)"=w1259, "Instrument in"=w1260) -> ("error out"=w1264:errorcluster, "ACK"=w1269:string, "Instrument out"=w1265:refnum<class "Inst.Krohn-Hite-7008.lvclass">)  [unwired: 7 in]
          n548 = case shown="\"\"" w1269 {
            tunnel: [w1273 w1281] -> w1268
            tunnel: w1266 -> [w1273 w1281]
            tunnel: [w1270 "" ("State(s) in Front (\"\")")] -> w1267
            tunnel: w1265 -> [w1272 w1279]
            tunnel: w1264 -> [w1271 w1278]
            tunnel: [w1271 w1277] -> w1263
            tunnel: [w1272 w1276] -> w1262
            tunnel: [w1270 w1274] -> w1256
            frame "" {
              w1270 = "" ("State(s) in Front (\"\")")
            }
            frame Default {
              n549 = call <userlib>:"IDN.vi"("error in (no error)"=w1278, "Instrument in"=w1279) -> ("error out"=w1277:errorcluster, "IDN"=w1275:T33, "Instrument in"=w1276:refnum<class "Inst.Krohn-Hite-7008.lvclass">)  [unwired: 7 in]
              n550 = Unbundle By Name(w1275) -> ("serial"=w1274:string)
            }
          }
          n551 = call-dynamic "Close.vi"("error in (no error)"=w1263, "Inst.Krohn-Hite-7008 in"=w1262) -> ()  [unwired: 8 in, 2 out]
        }
        n552 = call <vilib>:"1D String Array to Delimited String.vi"("delimiter"=",", "string array"=w1242) -> ("delimited string"=→"KH S/N":string)  [unwired: 9 in]
        n553 = Bundle By Name(cluster=w1250, "C.E."=w1249) -> (w1251:T23)
        n554 = call <vilib>:"Add State(s) to Queue__jki_lib_state_machine.vi"("State(s) in Front (\"\")"=w1248, "State(s) in (\"\")"=w1255) -> ("States Out"=w1254:string)  [unwired: 13 in]
      }
      frame "Instrument: Open Lockin" {
        n555 = call "Open Lockin.vi"("error in (no error)"=w1284) -> ("error out"=w1283:errorcluster)  [unwired: 10 in]
        n556 = call <vilib>:"Add State(s) to Queue__jki_lib_state_machine.vi"("State(s) in (\"\")"=w1287) -> ("States Out"=w1286:string)  [unwired: 14 in]
      }
      frame "Instrument: Open KH7008" {
        n557 = call "Open KH7008.vi"("error in (no error)"=w1290) -> ("error out"=w1289:errorcluster)  [unwired: 10 in]
        n558 = call <vilib>:"Add State(s) to Queue__jki_lib_state_machine.vi"("State(s) in (\"\")"=w1293) -> ("States Out"=w1292:string)  [unwired: 14 in]
      }
      frame "---------- Transport Server ----------" {
        # "Do not put any code in this frame.\n(it is a separator no-op)"
        n559 = call <vilib>:"Add State(s) to Queue__jki_lib_state_machine.vi"("State(s) in (\"\")"=w1298) -> ("States Out"=w1297:string)  [unwired: 14 in]
      }
      frame "Transport Server: Create" {
        n560 = Unbundle By Name(w1306) -> ("Transport-Server"=w1304:refnum<class "Inst.Transport.lvclass">)
        n561 = call <userlib>:"Create Instrument SMO.vi"("error in (no error)"=w1302, "Debug Mode? [F]"=FALSE, "Configuration Window? [T]"=FALSE, "Instrument in"=w1304) -> ("error out"=w1300:errorcluster, "Instrument out"=w1303:refnum<class "Inst.Transport.lvclass">)  [unwired: 6 in]
        n562 = Bundle By Name(cluster=w1306, "Transport-Server"=w1303) -> (w1307:T23)
        n563 = call <vilib>:"Add State(s) to Queue__jki_lib_state_machine.vi"("State(s) in (\"\")"=w1309) -> ("States Out"=w1308:string)  [unwired: 14 in]
      }
      frame "Transport Server: Start" {
        n564 = Unbundle By Name(w1311) -> ("Transport-Server"=w1316:refnum<class "Inst.Transport.lvclass">)
        n565 = call <vilib>:"Start.vi"("error in (no error)"=w1313, "SMO"=w1316) -> ("error out"=w1314:errorcluster, "SMO out"=w1315:refnum<class "Inst.Transport.lvclass">)  [unwired: 8 in]
        n566 = Bundle By Name(cluster=w1311, "Transport-Server"=w1315) -> (w1312:T23)
        n567 = call <vilib>:"Add State(s) to Queue__jki_lib_state_machine.vi"("State(s) in (\"\")"=w1318) -> ("States Out"=w1317:string)  [unwired: 14 in]
      }
      frame "Transport Server: Stop" {
        n568 = Unbundle By Name(w1323) -> ("Transport-Server"=w1321:refnum<class "Inst.Transport.lvclass">)
        n569 = call <vilib>:"Stop.vi"("error in (no error)"=w1320, "SMO"=w1321) -> ("error out"=w1319:errorcluster, "SMO out"=w1325:refnum<class "Inst.Transport.lvclass">)  [unwired: 8 in]
        n570 = Bundle By Name(cluster=w1323, "Transport-Server"=w1325) -> (w1324:T23)
        n571 = call <vilib>:"Add State(s) to Queue__jki_lib_state_machine.vi"("State(s) in (\"\")"=w1327) -> ("States Out"=w1326:string)  [unwired: 14 in]
      }
      frame "Transport Server: Destroy" {
        n572 = Unbundle By Name(w1330) -> ("Transport-Server"=w1334:refnum<class "Inst.Transport.lvclass">)
        n573 = call <vilib>:"Destroy.vi"("error in (no error)"=w1332, "SMO"=w1334) -> ("error out"=w1333:errorcluster)  [unwired: 9 in]
        n574 = Bundle By Name(cluster=w1330, "Transport-Server"=refnum<class "Inst.Transport.lvclass"> refnum ("Inst.Transport")) -> (w1331:T23)
        n575 = call <vilib>:"Add State(s) to Queue__jki_lib_state_machine.vi"("State(s) in (\"\")"=w1336) -> ("States Out"=w1335:string)  [unwired: 14 in]
      }
      frame "Transport Server: Show" {
        # "Do not put any code in this frame.\n(it is a separator no-op)"
        n576 = Unbundle By Name(w1341) -> ("Transport-Server"=w1337:refnum<class "Inst.Transport.lvclass">)
        n577 = call "showUI.vi"("error in (no error)"=w1339, "Inst.Transport in"=w1337) -> ("error out"=w1340:errorcluster)  [unwired: 8 in, 1 out]
        n578 = Bundle By Name(cluster=w1341, "Transport-Server"=w1337) -> (w1342:T23)
        n579 = call <vilib>:"Add State(s) to Queue__jki_lib_state_machine.vi"("State(s) in (\"\")"=w1344) -> ("States Out"=w1343:string)  [unwired: 14 in]
      }
      frame "Transport Server: Hide" {
        # "Do not put any code in this frame.\n(it is a separator no-op)"
        n580 = Unbundle By Name(w1349) -> ("Transport-Server"=w1345:refnum<class "Inst.Transport.lvclass">)
        n581 = call "hideUI.vi"("error in (no error)"=w1347, "Inst.Transport in"=w1345) -> ("error out"=w1348:errorcluster)  [unwired: 8 in, 1 out]
        n582 = Bundle By Name(cluster=w1349, "Transport-Server"=w1345) -> (w1350:T23)
        n583 = call <vilib>:"Add State(s) to Queue__jki_lib_state_machine.vi"("State(s) in (\"\")"=w1352) -> ("States Out"=w1351:string)  [unwired: 14 in]
      }
      frame "---------- PGSQL ----------" {
        # "Do not put any code in this frame.\n(it is a separator no-op)"
        n584 = call <vilib>:"Add State(s) to Queue__jki_lib_state_machine.vi"("State(s) in (\"\")"=w1357) -> ("States Out"=w1356:string)  [unwired: 14 in]
      }
      frame "PGSQL: Write" {
        w1368 = "" ("f")
        n585 = Unbundle By Name(w1371) -> ("Experiment.Device"=w1360:string, "Experiment.User"=w1370:string, "Experiment.Instrument"=w1369:string)
        n586 = local read "I'm Finished Taking Data!"() -> (w1361:bool)
        n587 = Not(x=w1361) -> (.not. x?=w1367:bool)
        n588 = Select(t=w1370, s=w1367, f=w1368) -> (s? t:f=w1365:string)
        n589 = Select(t=w1369, s=w1367, f=w1368) -> (s? t:f=w1366:string)
        n590 = local read "MCL S/N"() -> (w1359:string)
        n591 = local read "KH S/N"() -> (w1358:string)
        n592 = call "DB Set Measurement.vi"("KH serial number"=w1358, "lockin serial number"=w1359, "device"=w1360, "error in (no error)"=w1364, "Station"=w1366, "User"=w1365) -> ("error out"=w1363:errorcluster)  [unwired: 5 in]
        n593 = call <vilib>:"Add State(s) to Queue__jki_lib_state_machine.vi"("State(s) in (\"\")"=w1373) -> ("States Out"=w1372:string)  [unwired: 14 in]
      }
      frame "---------- Sequence ----------" {
        # "Do not put any code in this frame.\n(it is a separator no-op)"
        n594 = call <vilib>:"Add State(s) to Queue__jki_lib_state_machine.vi"("State(s) in (\"\")"=w1378) -> ("States Out"=w1377:string)  [unwired: 14 in]
      }
      frame "Sequence: Wait" {
        # "Do not put any code in this frame.\n(it is a separator no-op)"
        n595 = Scan From String(input string=w1381, default 1=u32 0 ("milliseconds to wait")) -> (output 1=w1380:u32)  [unwired: 3 in, 3 out]
        n596 = Wait (ms)(milliseconds to wait=w1380) -> ()  [unwired: 1 out]
        n597 = call <vilib>:"Add State(s) to Queue__jki_lib_state_machine.vi"("State(s) in (\"\")"=w1386) -> ("States Out"=w1385:string)  [unwired: 14 in]
      }
    }
  }
  "Error Out" <- w2
  n598 = Unbundle By Name(w6) -> ("C.E."=→"Control Experiment":refnum<class "Control Experiment.lvclass">)
